vi "ReadBinaryCore.vi"(7 "UpperLevelControlRefs.":T1, 9 "metadata in":refnum<queue>, 10 "data out in":refnum<queue>, 11 "Control Queue in":refnum<queue>) -> ()   [LabVIEW 2013]
uses:
  _BinaryFileViewer/ReaderUpperLevelRefs.ctl
  _BinaryFileViewer/BinaryReader_Params.ctl
  ControlDef/ProcessingMode.ctl
  _BinaryFileViewer/BinaryRead_State.ctl
  Signal_Segment.ctl
  BinaryHeader.ctl
  Signal_Segment_v3.ctl
  Signal_Segment_v35.ctl
  Signal_Segment_v36.ctl
  _FileFormatConversion/UIC-DepthProfileFormat/DepthProfileFileHeader.ctl
  _FileFormatConversion/UIC-DepthProfileFormat/DepthProfileFormat_Spectrum.ctl
  <vilib>/Utility/error.llb/DialogType.ctl
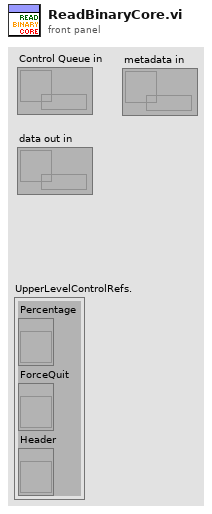
[diagram p1: front panel]
types:
  T1 = typedef "ReaderUpperLevelRefs.ctl" = cluster{"Percentage":refnum<vi>, "ForceQuit":refnum<vi>, "Header":refnum<vi>}
  T2 = typedef "BinaryReader_Params.ctl" = cluster{"FileVersion":string, "Start Position":dbl[], "StepWidth":dbl[], "Dimension":i32[], "TotalDepth":i32, "Spec#":u32, "FileSize":i64, "Calibr.":dbl[], "Position":dbl[], "Pressure":dbl, "Desp_LaserEnergy":dbl, "PI_LaserEnergy":dbl, "SpecLength":dbl, "Average#":i32, "SampleRate":dbl, "DAQ_Range":dbl, "Voltages Table":sgl[][], "ProcMode":T3, "Time Stamp":timestamp, "TrigDelay":dbl, "TickCount":dbl}
  T3 = typedef "ProcessingMode.ctl" = enum16{"None", "Drop by Threshold", "TDC Simulate", "SetFilter"}
  T4 = enum16{"open", "replace", "create", "open or create", "replace or create", "replace or create with confirmation"}
  T5 = typedef "Signal_Segment_v3.ctl" = cluster{"Signal":sgl[], "Calibr.":dbl[], "Position":dbl[], "Pressure":dbl, "Desp_LaserEnergy":dbl, "PI_LaserEnergy":dbl, "Depth":dbl, "Average":i32, "Acqu. Rate":dbl, "Voltages Table":sgl[][], "Acqu. Range":dbl, "Processing Mode":T3, "Threshold":dbl, "Comment":string, "Time Stamp":timestamp, "Operator":string}
  T6 = enum16{"big-endian, network order", "native, host order", "little-endian"}
  T7 = typedef "BinaryHeader.ctl" = cluster{"Start Position":dbl[], "StepWidth":dbl[], "Dimension":i32[], "SpecLength":i32}
  T8 = typedef "Signal_Segment_v35.ctl" = cluster{"SampleRate":dbl, "TrigDelay":dbl, "SpecLength":dbl, "DAQ_Range":dbl, "Average#":i32, "Position":dbl[], "Spectrum":sgl[], "Calibr.":dbl[], "Pressure":dbl, "Desp_LaserEnergy":dbl, "PI_LaserEnergy":dbl, "Voltages Table":sgl[][], "ProcMode":T3, "Threshold":dbl, "Comment":string, "Time Stamp":timestamp}
  T9 = typedef "Signal_Segment_v36.ctl" = cluster{"SampleRate":dbl, "TrigDelay":dbl, "SpecLength":dbl, "DAQ_Range":dbl, "Average#":i32, "Position":dbl[], "Spectrum":sgl[], "Calibr.":dbl[], "Pressure":dbl, "Desp_LaserEnergy":dbl, "PI_LaserEnergy":dbl, "Voltages Table":sgl[][], "ProcMode":T3, "Threshold":dbl, "Comment":string, "TickCount":dbl, "Time Stamp":timestamp}
  T10 = typedef "DepthProfileFormat_Spectrum.ctl" = cluster{"Average#":i16, "SpecLength":i32, "Spectrum":sgl[], "Cali.":dbl[], "Sample Rate":dbl}
  T11 = typedef "Signal_Segment.ctl" = cluster{"SampleRate":dbl, "TrigDelay":dbl, "SpecLength":dbl, "DAQ_Range":dbl, "Average#":i32, "Position":dbl[], "Spectrum":sgl[], "Calibr.":dbl[], "Pressure":dbl, "Desp_LaserEnergy":dbl, "PI_LaserEnergy":dbl, "Voltages Table":sgl[][], "ProcMode":T3, "Threshold":dbl, "Comment":string, "TickCount":dbl, "Time Stamp":timestamp}
  T12 = typedef "BinaryRead_State.ctl" = cluster{"State":enum16{"Open", "GetHeader", "Index", "Read_i", "Read_all", "Close", "Quit"}, "Params":variant}
  T13 = enum16{"Open", "GetHeader", "Index", "Read_i", "Read_all", "Close", "Quit"}
  T14 = typedef "DepthProfileFileHeader.ctl" = cluster{"SpecLength":i32, "Sample Rate":dbl, "Cali.":dbl[], "Total_Depth":i32}
  T15 = typedef "DialogType.ctl" = u16
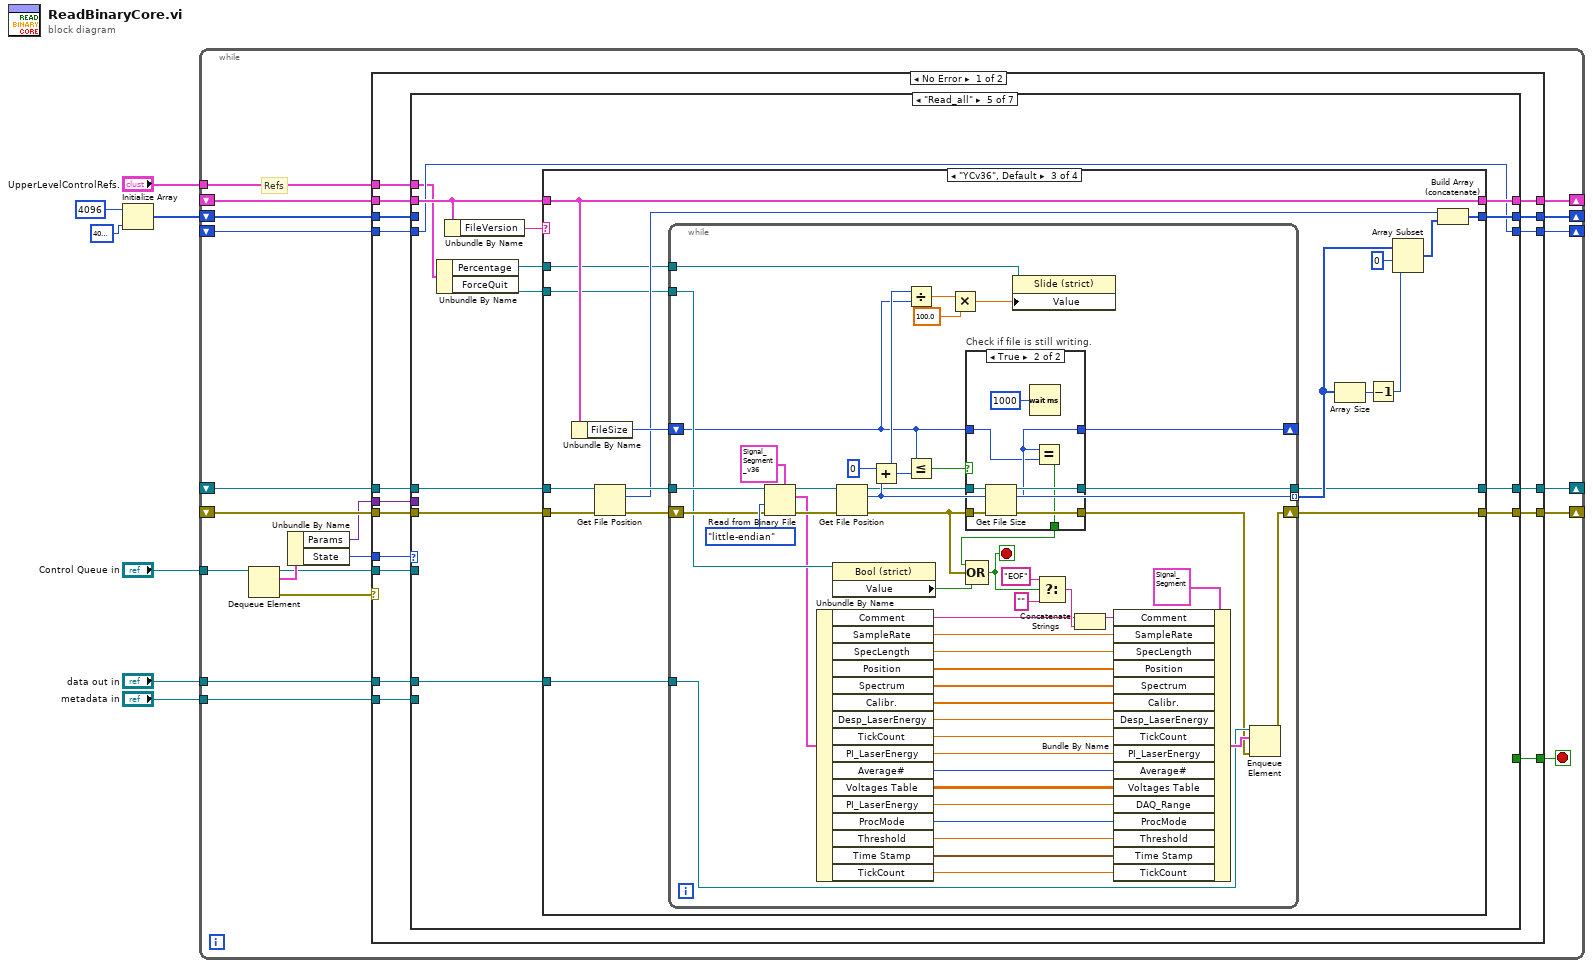
[diagram p0: block diagram]
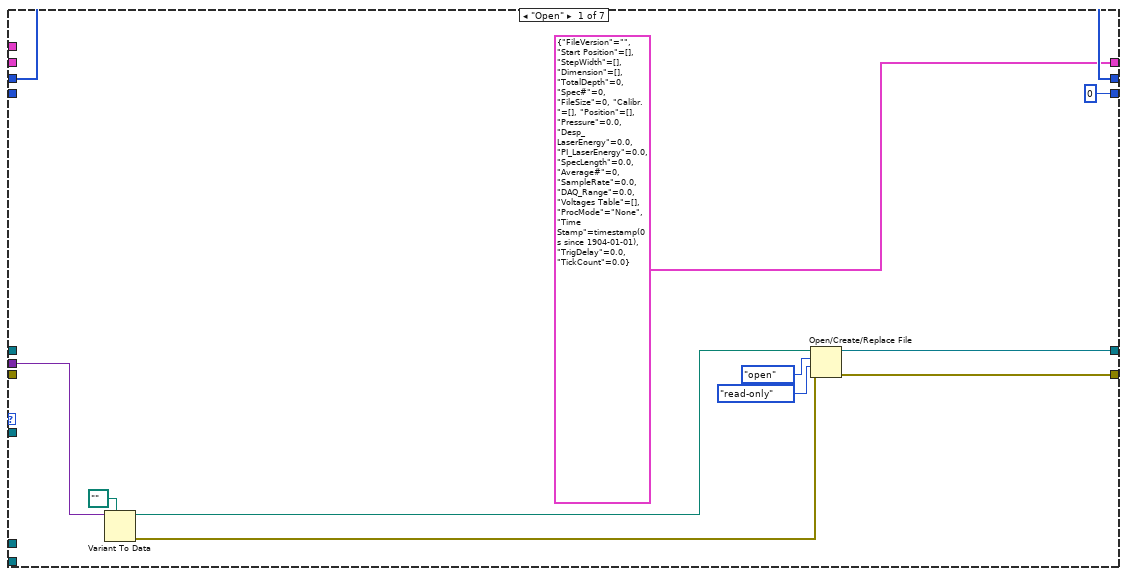
[diagram p2: hidden frame]
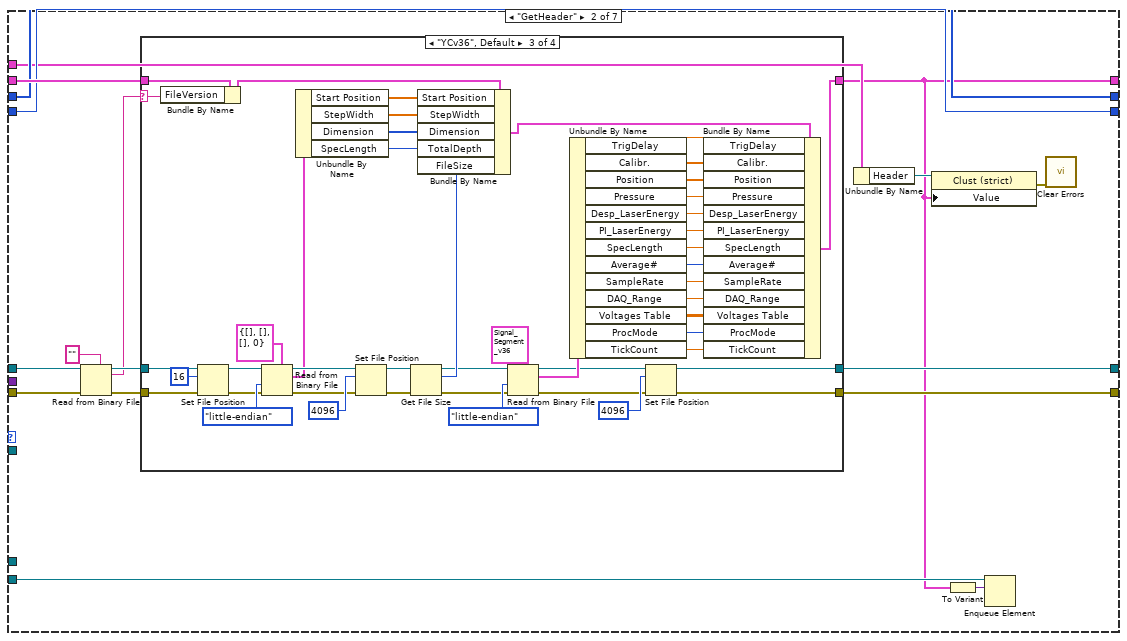
[diagram p3: hidden frame]
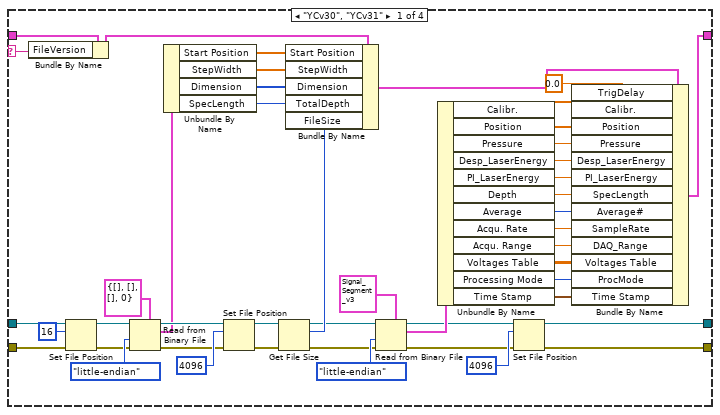
[diagram p4: hidden frame]
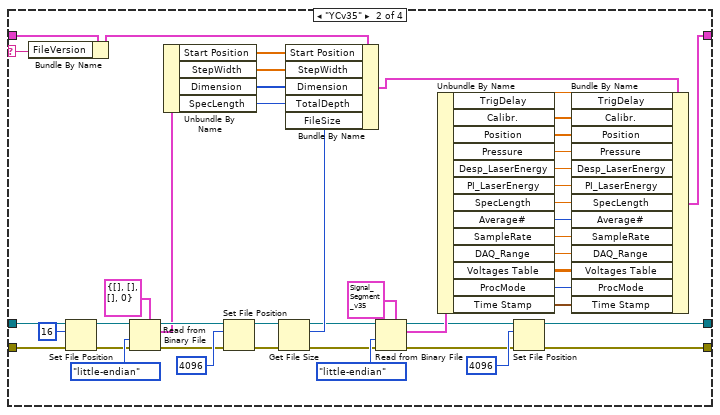
[diagram p5: hidden frame]
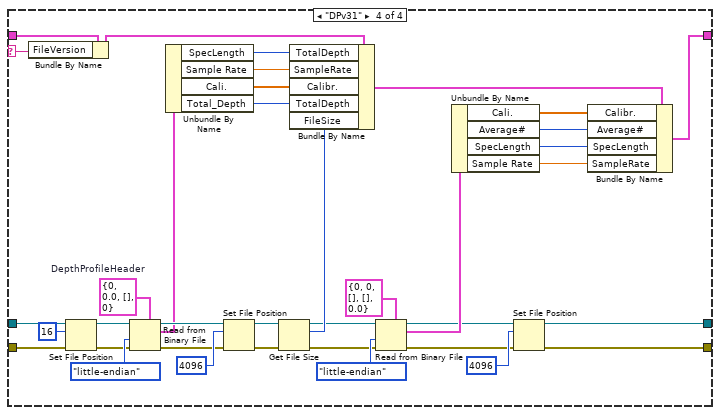
[diagram p6: hidden frame]
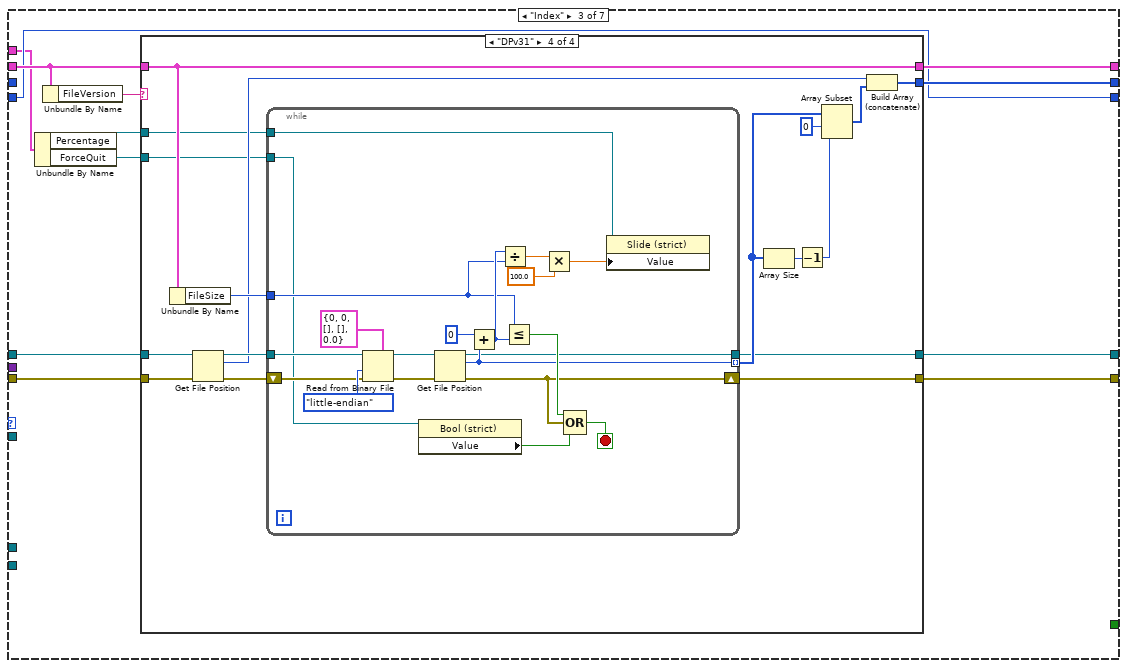
[diagram p7: hidden frame]
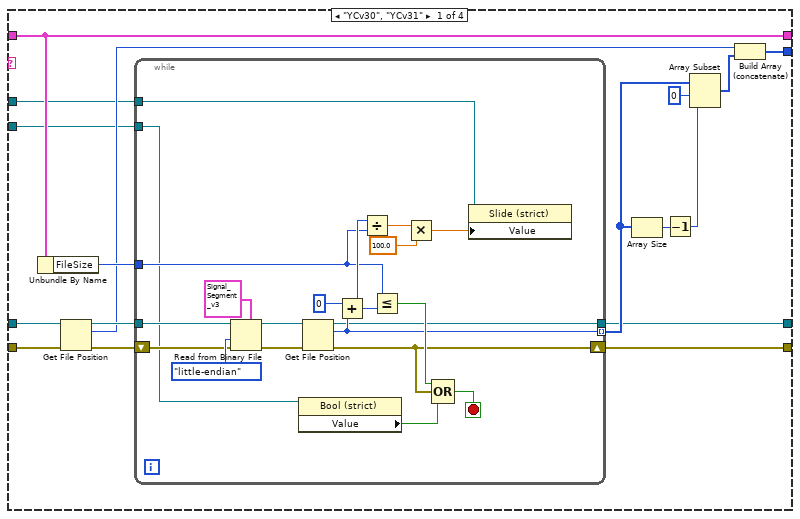
[diagram p8: hidden frame]
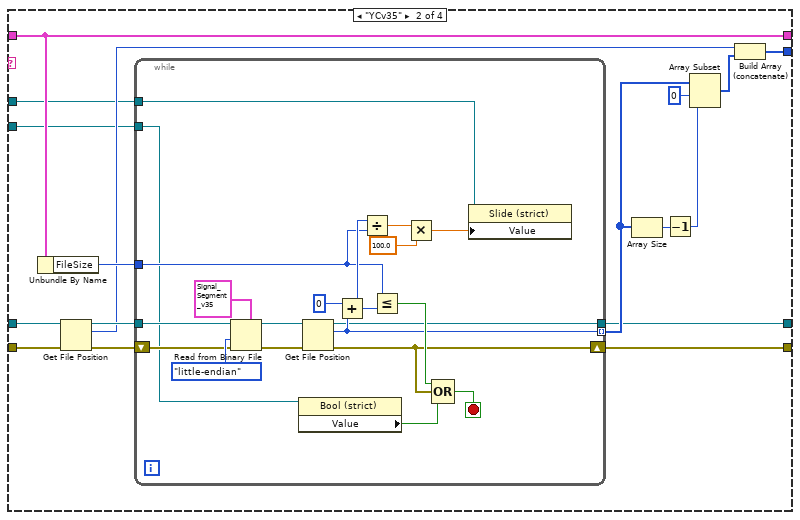
[diagram p9: hidden frame]
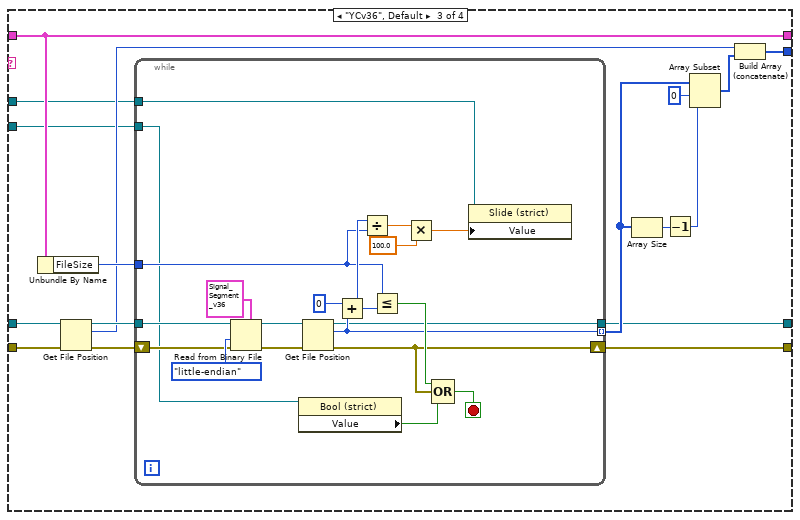
[diagram p10: hidden frame]
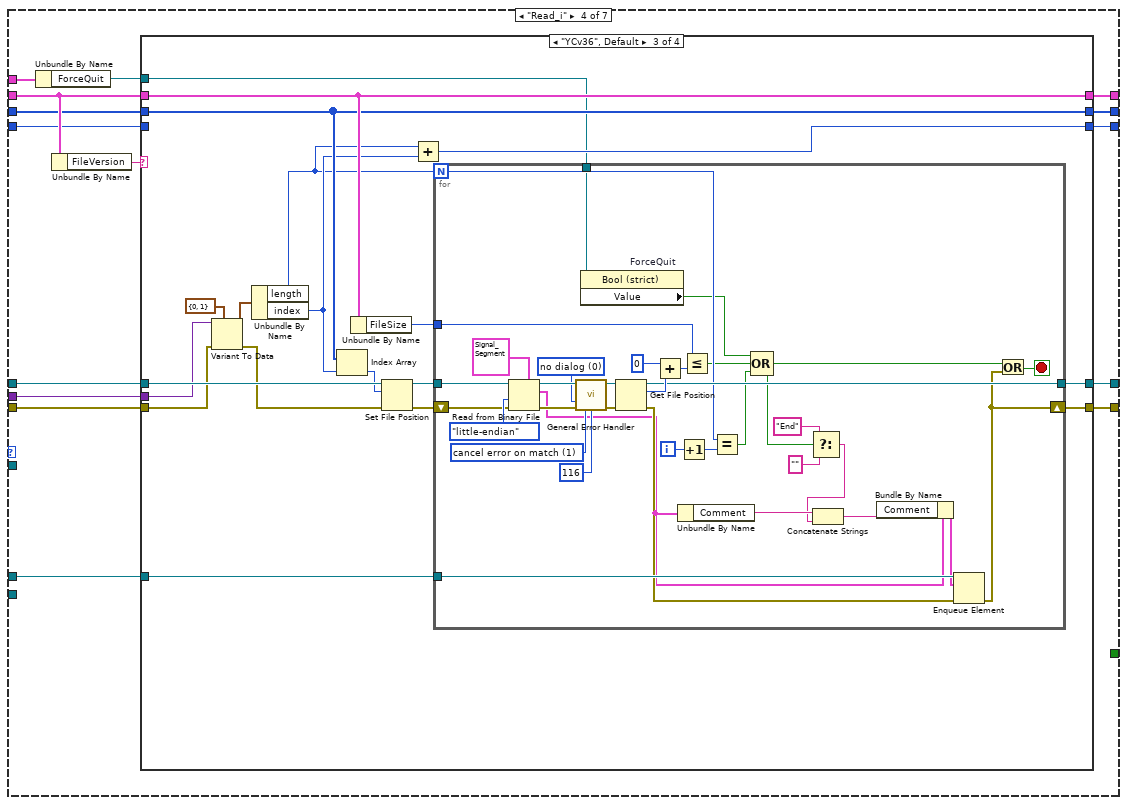
[diagram p11: hidden frame]
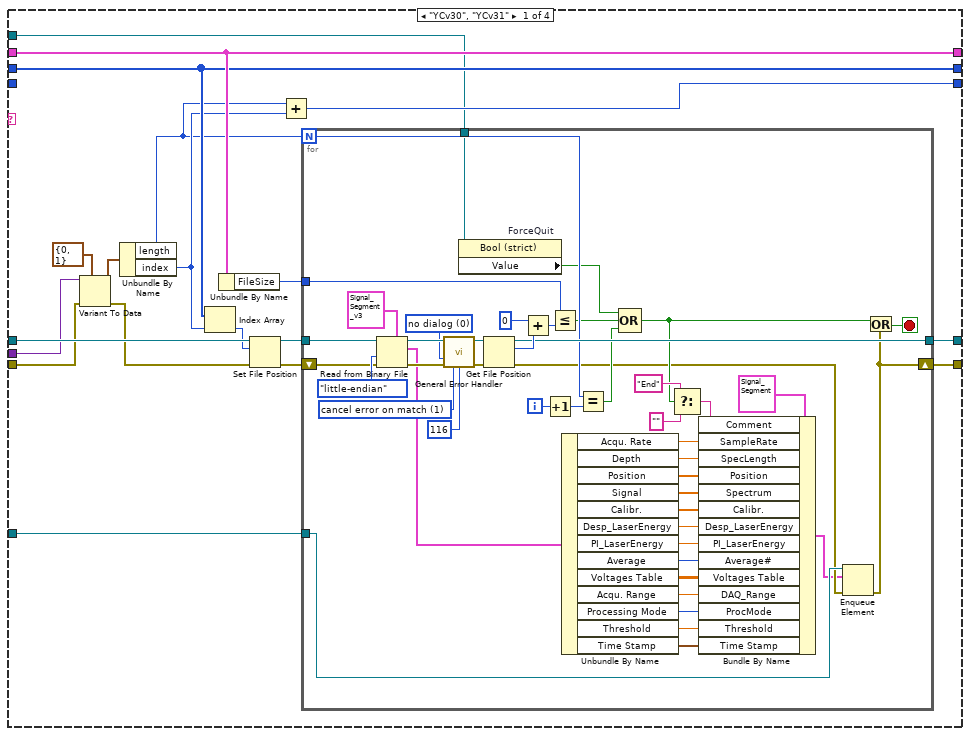
[diagram p12: hidden frame]
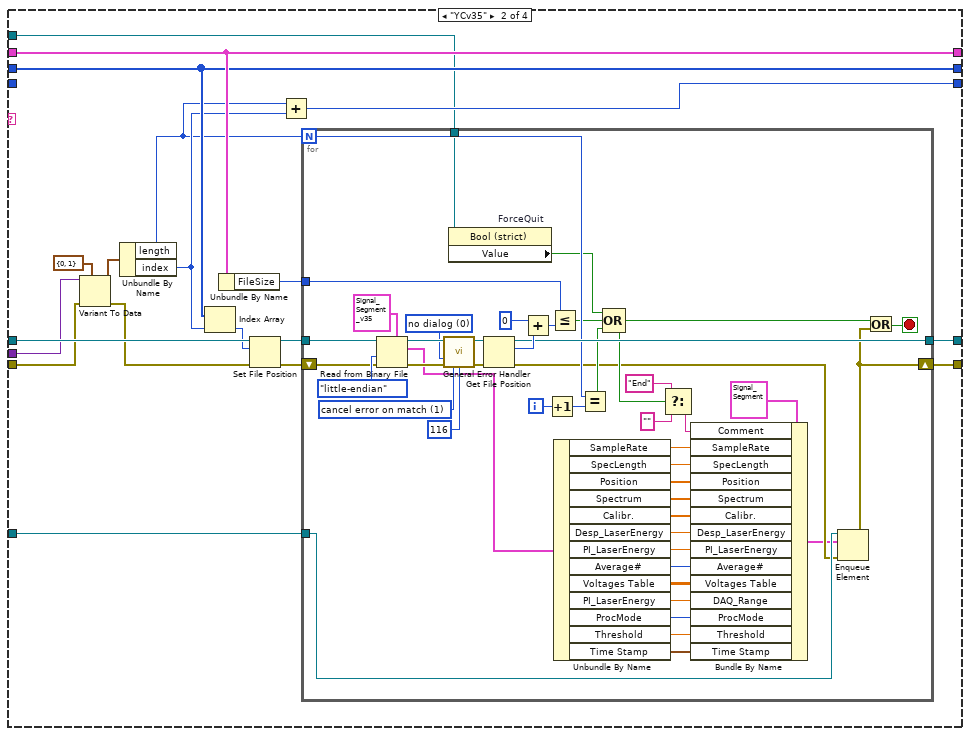
[diagram p13: hidden frame]
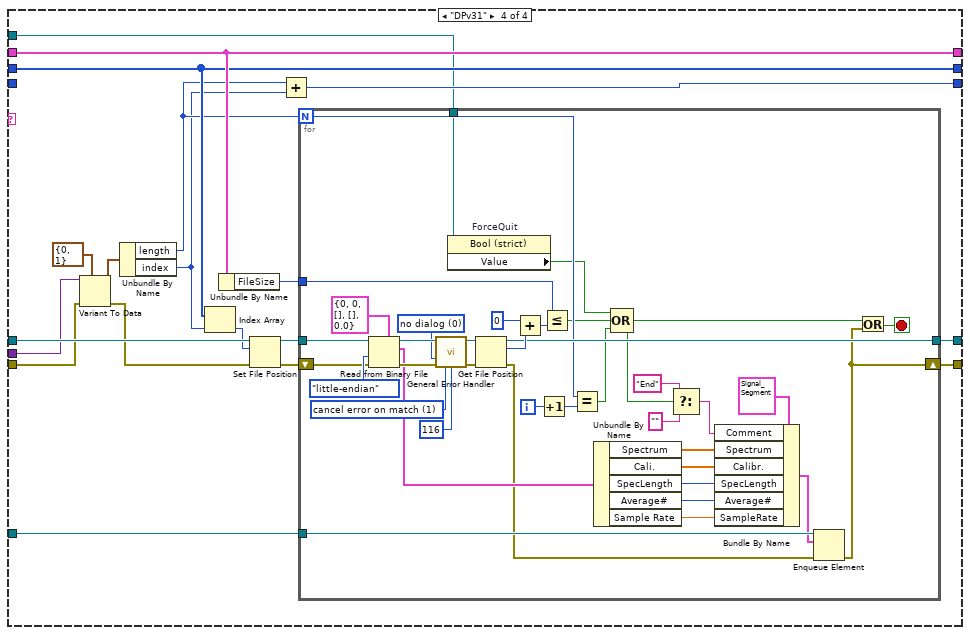
[diagram p14: hidden frame]
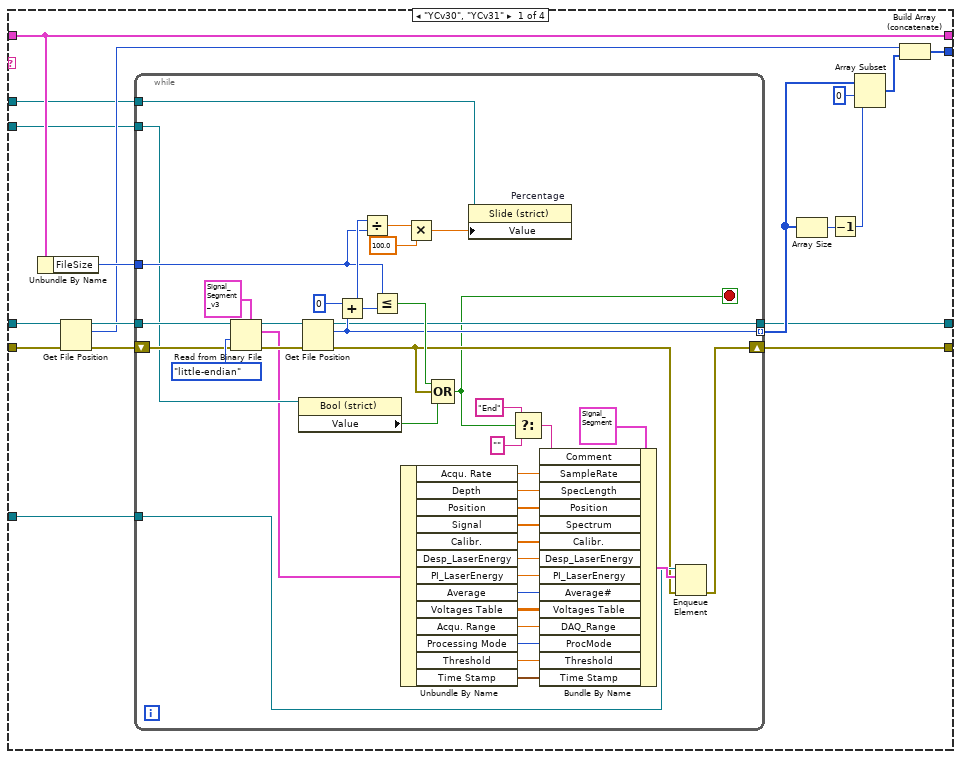
[diagram p15: hidden frame]
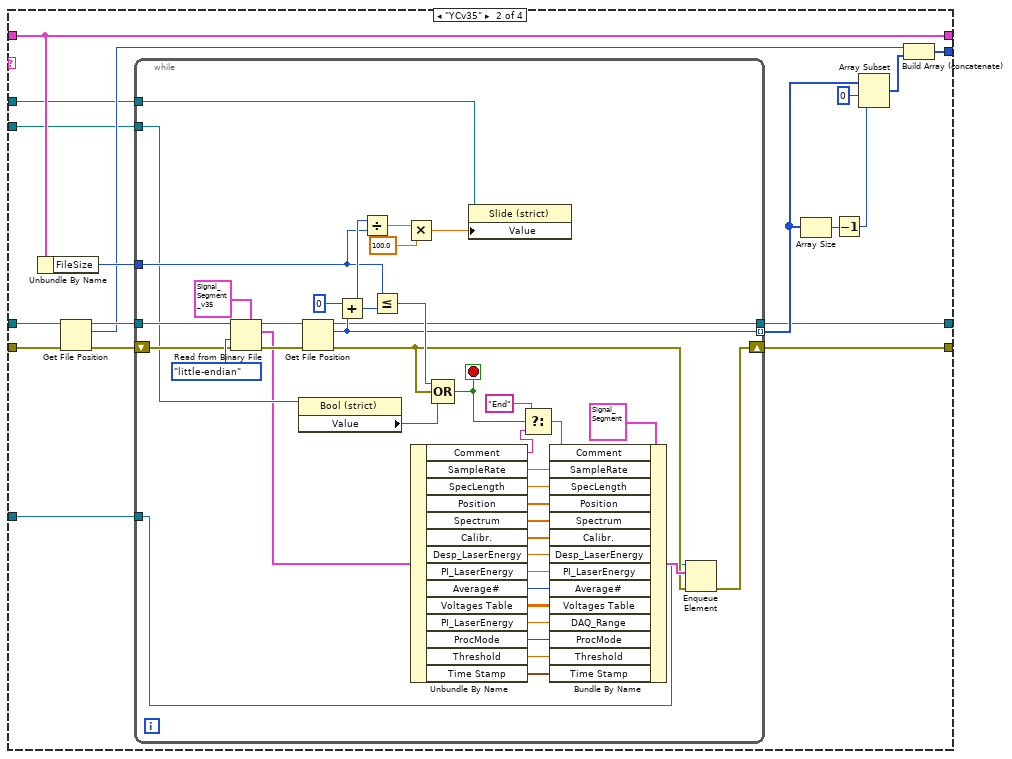
[diagram p16: hidden frame]
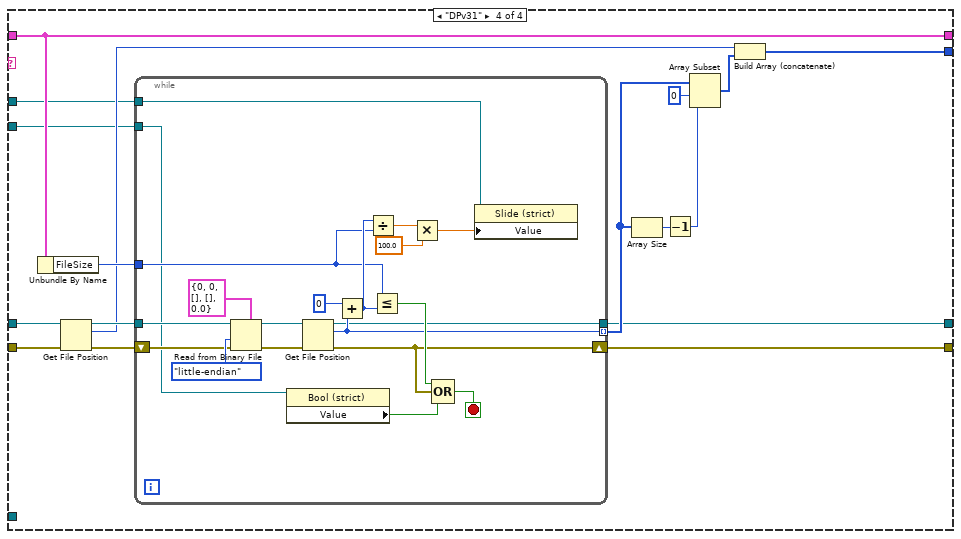
[diagram p18: hidden frame]
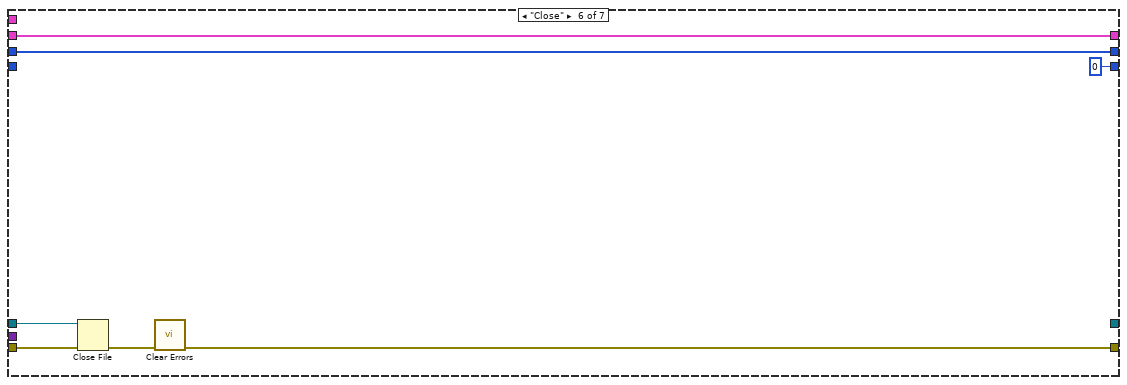
[diagram p19: hidden frame]
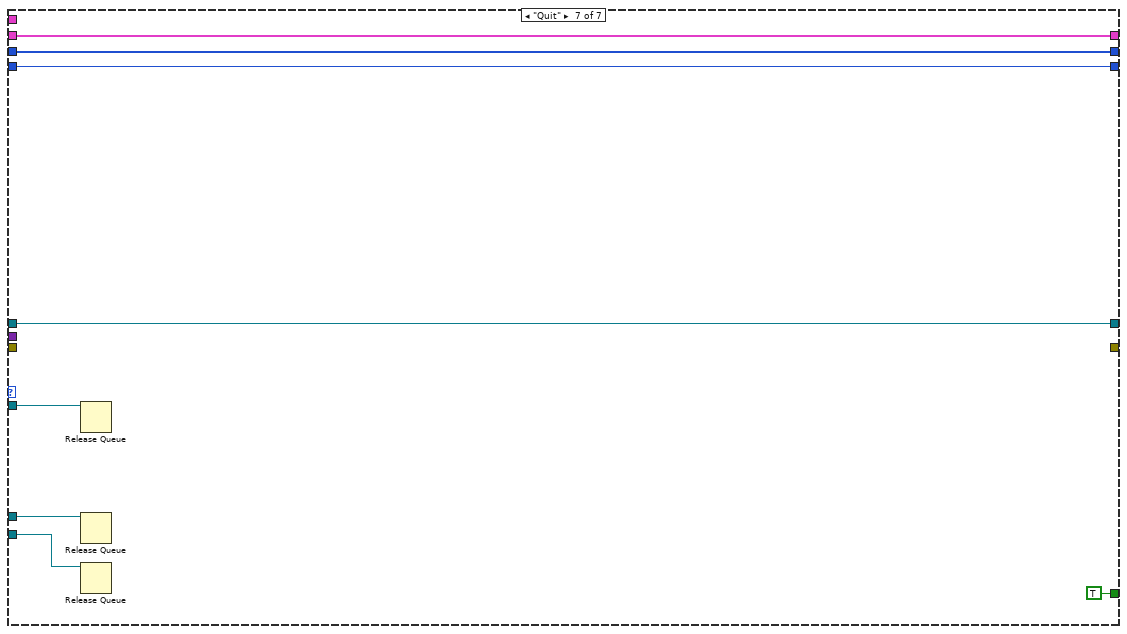
[diagram p20: hidden frame]
diagram:
  n1 = Initialize Array(i64 4096, 4000000 ("dimension size")) -> (w4:i64[])
  n2 = while {
    shift-right: [w26] -> _
    shift-left: _ -> [w27]
    shift-right: [w25] -> _
    shift-left: _ -> [w24]
    shift-right: [w23] -> _
    shift-left: _ -> [w22]
    shift-right: [w20] -> _
    shift-left: w4 -> [w21]
    tunnel: "data out in" -> [w19]
    shift-right: [w17] -> _
    shift-left: _ -> [w18]
    tunnel: "Control Queue in" -> [w16]
    tunnel: "UpperLevelControlRefs." -> [w10]
    tunnel: "metadata in" -> [w9]
    stop <- w11 stop-if-true
    # "Refs"
    n3 = Dequeue Element(queue=w16) -> (queue out=w8:refnum<queue>, element=w15:T12, error out=w12:errorcluster)  [unwired: 2 in, 1 out]
    n4 = Unbundle By Name(w15) -> ("Params"=w13:variant, "State"=w14:T13)
    n5 = case shown="No Error" w12 {
      tunnel: w27 -> [w44 w925]
      tunnel: [w43 w925] -> w26
      tunnel: [w42 w926] -> w25
      tunnel: w24 -> [w41 w926]
      tunnel: [w40 w929] -> w23
      tunnel: w22 -> [w39 w929]
      tunnel: w21 -> [w38 w928]
      tunnel: [w37 w928] -> w20
      tunnel: w19 -> [w36 _]
      tunnel: w18 -> [w35 w927]
      tunnel: [w34 w927] -> w17
      tunnel: w14 -> [w33 _]
      tunnel: w13 -> [w32 _]
      tunnel: [w31 TRUE] -> w11
      tunnel: w10 -> [w30 _]
      tunnel: w9 -> [w29 _]
      tunnel: w8 -> [w28 _]
      frame No Error {
        n6 = case shown="\"Read_all\"" w33 {
          tunnel: w44 -> [_ w72 w255 w419 w671 w911 _]
          tunnel: [w46 w66 w259 w410 w675 w910 _] -> w43
          tunnel: [w47 w65 w258 w422 w674 _ w923] -> w42
          tunnel: w41 -> [_ w69 w256 w420 w672 w915 w923]
          tunnel: [T2 {"FileVersion"="", "Start Position"=[], "StepWidth"=[], "Dimension"=[], "TotalDepth"=0, "Spec#"=0, "FileSize"=0, "Calibr."=[], "Position"=[], "Pressure"=0.0, "Desp_LaserEnergy"=0.0, "PI_LaserEnergy"=0.0, "SpecLength"=0.0, "Average#"=0, "SampleRate"=0.0, "DAQ_Range"=0.0, "Voltages Table"=[], "ProcMode"=enum."None", "Time Stamp"=timestamp(0 s since 1904-01-01), "TrigDelay"=0.0, "TickCount"=0.0} ("Header") w56 w257 w421 w673 w914 w922] -> w40
          tunnel: w39 -> [_ w64 w254 w418 w670 w914 w922]
          tunnel: w38 -> [w48 w63 _ w415 _ w913 w921]
          tunnel: [w48 w63 w252 w416 w668 w913 w921] -> w37
          tunnel: w32 -> [w52 _ _ w414 _ _ _]
          tunnel: w36 -> [_ _ _ w413 w663 _ w919]
          tunnel: w35 -> [_ w62 w251 w412 w667 _ w920]
          tunnel: [0 ("index") w62 w251 w411 w667 0 ("index") w920] -> w34
          tunnel: [_ _ _ _ _ _ TRUE] -> w31
          tunnel: w30 -> [_ w61 w250 w409 w666 _ _]
          tunnel: w29 -> [_ w59 _ _ _ _ w917]
          tunnel: w28 -> [_ _ _ _ _ _ w916]
          frame "Open" {
            n7 = Variant To Data(type=path "" ("file path (use dialog)"), Variant=w52) -> (data=w51:path, error out=w50:errorcluster)  [unwired: 1 in]
            n8 = Open/Create/Replace File(file path (use dialog)=w51, error in=w50, operation (0:open)=T4."open", access (0:read/write)=enum16{"read/write", "read-only", "write-only"}."read-only") -> (refnum out=w47:refnum<file>, error out=w46:errorcluster)  [unwired: 2 in, 1 out]
          }
          frame "GetHeader" {
            n9 = Read from Binary File(5:"" ("data type"), 8:w72, 11:w69) -> (0:w71:errorcluster, 2:w68:string, 3:w70:refnum<file>)  [unwired: 3 in, 1 out]
            n10 = case shown="\"YCv36\", Default" w68 {
              selector: w68 -> [w100 w146 w192 w230]
              tunnel: w71 -> [w113 w159 w205 w243]
              tunnel: w70 -> [w112 w158 w204 w242]
              tunnel: [w75 w122 w168 w215] -> w66
              tunnel: [w76 w123 w169 w216] -> w65
              tunnel: [w91 w137 w183 w222] -> w56
              tunnel: w64 -> [w108 w154 w200 w238]
              frame "YCv30", "YCv31" {
                n11 = Bundle By Name(cluster=w108, "FileVersion"=w100) -> (w101:T2)
                n12 = Set File Position(offset (in bytes) (0)=i64 16, refnum=w112, error in=w113) -> (refnum out=w116:refnum<file>, error out=w114:errorcluster)  [unwired: 1 in]
                n13 = Read from Binary File(5:T7 {"Start Position"=[], "StepWidth"=[], "Dimension"=[], "SpecLength"=0} ("File Header"), 8:w114, 9:T6."little-endian" ("byte order (0:big-endian, network order)"), 11:w116) -> (0:w96:errorcluster, 2:w106:T7, 3:w110:refnum<file>)  [unwired: 2 in, 1 out]
                n14 = Unbundle By Name(w106) -> ("Start Position"=w105:dbl[], "StepWidth"=w104:dbl[], "Dimension"=w103:i32[], "SpecLength"=w102:i32)
                n15 = Set File Position(offset (in bytes) (0)=i64 4096, refnum=w110, error in=w96) -> (refnum out=w111:refnum<file>, error out=w95:errorcluster)  [unwired: 1 in]
                n16 = Get File Size(file=w111, error in=w95) -> (refnum out=w93:refnum<file>, size (in bytes)=w99:i64, 0:w94:errorcluster)
                n17 = Bundle By Name(cluster=w101, "Start Position"=w105, "StepWidth"=w104, "Dimension"=w103, "TotalDepth"=w102, "FileSize"=w99) -> (w107:T2)
                n18 = Read from Binary File(5:T5 {"Signal"=[], "Calibr."=[], "Position"=[], "Pressure"=0.0, "Desp_LaserEnergy"=0.05, "PI_LaserEnergy"=0.05, "Depth"=0.0, "Average"=0, "Acqu. Rate"=0.0, "Voltages Table"=[], "Acqu. Range"=0.0, "Processing Mode"=enum."None", "Threshold"=0.05, "Comment"="", "Time Stamp"=timestamp(0 s since 1904-01-01), "Operator"=""} ("Signal Segment"), 8:w94, 9:T6."little-endian" ("byte order (0:big-endian, network order)"), 11:w93) -> (0:w74:errorcluster, 2:w92:T5, 3:w77:refnum<file>)  [unwired: 2 in, 1 out]
                n19 = Unbundle By Name(w92) -> ("Calibr."=w90:dbl[], "Position"=w89:dbl[], "Pressure"=w88:dbl, "Desp_LaserEnergy"=w87:dbl, "PI_LaserEnergy"=w86:dbl, "Depth"=w85:dbl, "Average"=w84:i32, "Acqu. Rate"=w83:dbl, "Acqu. Range"=w82:dbl, "Voltages Table"=w81:sgl[][], "Processing Mode"=w80:T3, "Time Stamp"=w79:timestamp)
                n20 = Set File Position(offset (in bytes) (0)=i64 4096, refnum=w77, error in=w74) -> (refnum out=w76:refnum<file>, error out=w75:errorcluster)  [unwired: 1 in]
                n21 = Bundle By Name(cluster=w107, "TrigDelay"=0.0, "Calibr."=w90, "Position"=w89, "Pressure"=w88, "Desp_LaserEnergy"=w87, "PI_LaserEnergy"=w86, "SpecLength"=w85, "Average#"=w84, "SampleRate"=w83, "DAQ_Range"=w82, "Voltages Table"=w81, "ProcMode"=w80, "Time Stamp"=w79) -> (w91:T2)
              }
              frame "YCv35" {
                n22 = Bundle By Name(cluster=w154, "FileVersion"=w146) -> (w147:T2)
                n23 = Set File Position(offset (in bytes) (0)=i64 16, refnum=w158, error in=w159) -> (refnum out=w162:refnum<file>, error out=w160:errorcluster)  [unwired: 1 in]
                n24 = Read from Binary File(5:T7 {"Start Position"=[], "StepWidth"=[], "Dimension"=[], "SpecLength"=0} ("File Header"), 8:w160, 9:T6."little-endian" ("byte order (0:big-endian, network order)"), 11:w162) -> (0:w142:errorcluster, 2:w152:T7, 3:w156:refnum<file>)  [unwired: 2 in, 1 out]
                n25 = Unbundle By Name(w152) -> ("Start Position"=w151:dbl[], "StepWidth"=w150:dbl[], "Dimension"=w149:i32[], "SpecLength"=w148:i32)
                n26 = Set File Position(offset (in bytes) (0)=i64 4096, refnum=w156, error in=w142) -> (refnum out=w157:refnum<file>, error out=w141:errorcluster)  [unwired: 1 in]
                n27 = Get File Size(file=w157, error in=w141) -> (refnum out=w139:refnum<file>, size (in bytes)=w145:i64, 0:w140:errorcluster)
                n28 = Bundle By Name(cluster=w147, "Start Position"=w151, "StepWidth"=w150, "Dimension"=w149, "TotalDepth"=w148, "FileSize"=w145) -> (w153:T2)
                n29 = Read from Binary File(5:T8 {"SampleRate"=0.0, "TrigDelay"=0.0, "SpecLength"=0.0, "DAQ_Range"=0.0, "Average#"=0, "Position"=[], "Spectrum"=[], "Calibr."=[], "Pressure"=0.0, "Desp_LaserEnergy"=0.0, "PI_LaserEnergy"=0.0, "Voltages Table"=[], "ProcMode"=enum."None", "Threshold"=0.0, "Comment"="", "Time Stamp"=timestamp(0 s since 1904-01-01)} ("Signal Segment"), 8:w140, 9:T6."little-endian" ("byte order (0:big-endian, network order)"), 11:w139) -> (0:w121:errorcluster, 2:w138:T8, 3:w124:refnum<file>)  [unwired: 2 in, 1 out]
                n30 = Unbundle By Name(w138) -> ("TrigDelay"=w120:dbl, "Calibr."=w136:dbl[], "Position"=w135:dbl[], "Pressure"=w134:dbl, "Desp_LaserEnergy"=w133:dbl, "PI_LaserEnergy"=w132:dbl, "SpecLength"=w131:dbl, "Average#"=w130:i32, "SampleRate"=w129:dbl, "DAQ_Range"=w128:dbl, "Voltages Table"=w127:sgl[][], "ProcMode"=w126:T3, "Time Stamp"=w119:timestamp)
                n31 = Set File Position(offset (in bytes) (0)=i64 4096, refnum=w124, error in=w121) -> (refnum out=w123:refnum<file>, error out=w122:errorcluster)  [unwired: 1 in]
                n32 = Bundle By Name(cluster=w153, "TrigDelay"=w120, "Calibr."=w136, "Position"=w135, "Pressure"=w134, "Desp_LaserEnergy"=w133, "PI_LaserEnergy"=w132, "SpecLength"=w131, "Average#"=w130, "SampleRate"=w129, "DAQ_Range"=w128, "Voltages Table"=w127, "ProcMode"=w126, "Time Stamp"=w119) -> (w137:T2)
              }
              frame "YCv36", Default {
                n33 = Bundle By Name(cluster=w200, "FileVersion"=w192) -> (w193:T2)
                n34 = Set File Position(offset (in bytes) (0)=i64 16, refnum=w204, error in=w205) -> (refnum out=w208:refnum<file>, error out=w206:errorcluster)  [unwired: 1 in]
                n35 = Read from Binary File(5:T7 {"Start Position"=[], "StepWidth"=[], "Dimension"=[], "SpecLength"=0} ("File Header"), 8:w206, 9:T6."little-endian" ("byte order (0:big-endian, network order)"), 11:w208) -> (0:w188:errorcluster, 2:w198:T7, 3:w202:refnum<file>)  [unwired: 2 in, 1 out]
                n36 = Unbundle By Name(w198) -> ("Start Position"=w197:dbl[], "StepWidth"=w196:dbl[], "Dimension"=w195:i32[], "SpecLength"=w194:i32)
                n37 = Set File Position(offset (in bytes) (0)=i64 4096, refnum=w202, error in=w188) -> (refnum out=w203:refnum<file>, error out=w187:errorcluster)  [unwired: 1 in]
                n38 = Get File Size(file=w203, error in=w187) -> (refnum out=w185:refnum<file>, size (in bytes)=w191:i64, 0:w186:errorcluster)
                n39 = Bundle By Name(cluster=w193, "Start Position"=w197, "StepWidth"=w196, "Dimension"=w195, "TotalDepth"=w194, "FileSize"=w191) -> (w199:T2)
                n40 = Read from Binary File(5:T9 {"SampleRate"=-1.0, "TrigDelay"=0.0, "SpecLength"=0.0, "DAQ_Range"=0.0, "Average#"=0, "Position"=[], "Spectrum"=[], "Calibr."=[], "Pressure"=-1.0, "Desp_LaserEnergy"=-1.0, "PI_LaserEnergy"=-1.0, "Voltages Table"=[], "ProcMode"=enum."None", "Threshold"=-1.0, "Comment"="", "TickCount"=0.0, "Time Stamp"=timestamp(0 s since 1904-01-01)} ("Signal Segment"), 8:w186, 9:T6."little-endian" ("byte order (0:big-endian, network order)"), 11:w185) -> (0:w167:errorcluster, 2:w184:T9, 3:w170:refnum<file>)  [unwired: 2 in, 1 out]
                n41 = Unbundle By Name(w184) -> ("TrigDelay"=w166:dbl, "Calibr."=w182:dbl[], "Position"=w181:dbl[], "Pressure"=w180:dbl, "Desp_LaserEnergy"=w179:dbl, "PI_LaserEnergy"=w178:dbl, "SpecLength"=w177:dbl, "Average#"=w176:i32, "SampleRate"=w175:dbl, "DAQ_Range"=w174:dbl, "Voltages Table"=w173:sgl[][], "ProcMode"=w172:T3, "TickCount"=w165:dbl)
                n42 = Set File Position(offset (in bytes) (0)=i64 4096, refnum=w170, error in=w167) -> (refnum out=w169:refnum<file>, error out=w168:errorcluster)  [unwired: 1 in]
                n43 = Bundle By Name(cluster=w199, "TrigDelay"=w166, "Calibr."=w182, "Position"=w181, "Pressure"=w180, "Desp_LaserEnergy"=w179, "PI_LaserEnergy"=w178, "SpecLength"=w177, "Average#"=w176, "SampleRate"=w175, "DAQ_Range"=w174, "Voltages Table"=w173, "ProcMode"=w172, "TickCount"=w165) -> (w183:T2)
              }
              frame "DPv31" {
                w213 = T14 {"SpecLength"=0, "Sample Rate"=0.0, "Cali."=[], "Total_Depth"=0}  # DepthProfileHeader
                n44 = Bundle By Name(cluster=w238, "FileVersion"=w230) -> (w231:T2)
                n45 = Set File Position(offset (in bytes) (0)=i64 16, refnum=w242, error in=w243) -> (refnum out=w246:refnum<file>, error out=w244:errorcluster)  [unwired: 1 in]
                n46 = Read from Binary File(5:w213, 8:w244, 9:T6."little-endian" ("byte order (0:big-endian, network order)"), 11:w246) -> (0:w227:errorcluster, 2:w236:T14, 3:w240:refnum<file>)  [unwired: 2 in, 1 out]
                n47 = Unbundle By Name(w236) -> ("SpecLength"=w235:i32, "Sample Rate"=w234:dbl, "Cali."=w233:dbl[], "Total_Depth"=w232:i32)
                n48 = Set File Position(offset (in bytes) (0)=i64 4096, refnum=w240, error in=w227) -> (refnum out=w241:refnum<file>, error out=w226:errorcluster)  [unwired: 1 in]
                n49 = Get File Size(file=w241, error in=w226) -> (refnum out=w224:refnum<file>, size (in bytes)=w229:i64, 0:w225:errorcluster)
                n50 = Bundle By Name(cluster=w231, "TotalDepth"=w235, "SampleRate"=w234, "Calibr."=w233, "TotalDepth"=w232, "FileSize"=w229) -> (w237:T2)
                n51 = Read from Binary File(5:T10 {"Average#"=0, "SpecLength"=0, "Spectrum"=[], "Cali."=[], "Sample Rate"=0.0} ("cluster"), 8:w225, 9:T6."little-endian" ("byte order (0:big-endian, network order)"), 11:w224) -> (0:w214:errorcluster, 2:w223:T10, 3:w217:refnum<file>)  [unwired: 2 in, 1 out]
                n52 = Unbundle By Name(w223) -> ("Cali."=w221:dbl[], "Average#"=w220:i16, "SpecLength"=w219:i32, "Sample Rate"=w211:dbl)
                n53 = Set File Position(offset (in bytes) (0)=i64 4096, refnum=w217, error in=w214) -> (refnum out=w216:refnum<file>, error out=w215:errorcluster)  [unwired: 1 in]
                n54 = Bundle By Name(cluster=w237, "Calibr."=w221, "Average#"=w220, "SpecLength"=w219, "SampleRate"=w211) -> (w222:T2)
              }
            }
            n55 = Unbundle By Name(w61) -> ("Header"=w60:refnum<vi>)
            n56 = property class="Clust (strict)"(reference=w60, "Value"=w56) -> (error out=w58:errorcluster)  [unwired: 1 in, 1 out]
            n57 = To Variant(anything=w56) -> (Variant=w57:variant)
            n58 = Enqueue Element(queue=w59, element=w57) -> ()  [unwired: 2 in, 3 out]
            n59 = call <vilib>:"Clear Errors.vi"("error in (no error)"=w58) -> ()  [unwired: 6 in, 1 out]
          }
          frame "Index" {
            n60 = Unbundle By Name(w250) -> ("Percentage"=w249:refnum<vi>, "ForceQuit"=w248:refnum<vi>)
            n61 = Unbundle By Name(w254) -> ("FileVersion"=w253:string)
            n62 = case shown="\"DPv31\"" w253 {
              tunnel: w255 -> [w275 w312 w349 w386]
              tunnel: w256 -> [w276 w313 w350 w387]
              tunnel: [w274 w311 w348 w385] -> w259
              tunnel: [w262 w299 w336 w373] -> w258
              tunnel: [w272 w309 w346 w383] -> w257
              tunnel: w254 -> [w272 w309 w346 w383]
              tunnel: [w269 w306 w343 w380] -> w252
              tunnel: w249 -> [w261 w298 w335 w372]
              tunnel: w248 -> [w260 w297 w334 w371]
              frame "YCv30", "YCv31" {
                n63 = Unbundle By Name(w272) -> ("FileSize"=w270:i64)
                n64 = Get File Position(4:w275, 7:w276) -> (0:w273:errorcluster, 2:w268:i64, 3:w271:refnum<file>)
                n65 = while {
                  tunnel: w271 -> [w290]
                  shift-right: [w287] -> w274
                  shift-left: w273 -> [w293]
                  tunnel: w270 -> [w279]
                  tunnel: [w286] -> w266 mode=indexing
                  tunnel: [w285] -> w262
                  tunnel: w261 -> [w281]
                  tunnel: w260 -> [w277]
                  stop <- w289 stop-if-true
                  n66 = Read from Binary File(5:T5 {"Signal"=[], "Calibr."=[], "Position"=[], "Pressure"=0.0, "Desp_LaserEnergy"=0.05, "PI_LaserEnergy"=0.05, "Depth"=0.0, "Average"=0, "Acqu. Rate"=0.0, "Voltages Table"=[], "Acqu. Range"=0.0, "Processing Mode"=enum."None", "Threshold"=0.05, "Comment"="", "Time Stamp"=timestamp(0 s since 1904-01-01), "Operator"=""} ("Signal Segment"), 8:w293, 9:T6."little-endian" ("byte order (0:big-endian, network order)"), 11:w290) -> (0:w294:errorcluster, 3:w291:refnum<file>)  [unwired: 2 in, 2 out]
                  n67 = property class="Bool (strict)"(reference=w277) -> ("Value"=w278:bool)  [unwired: 1 in, 2 out]
                  n68 = Get File Position(4:w294, 7:w291) -> (0:w287:errorcluster, 2:w286:i64, 3:w285:refnum<file>)
                  n69 = Add(x=i64 0, y=w286) -> (x+y=w280:i64)
                  n70 = Divide(x=w280, y=w279) -> (x/y=w283:dbl)
                  n71 = Less Or Equal?(x=w279, y=w280) -> (x <= y?=w288:bool)
                  n72 = Multiply(x=w283, y=100.0 ("x")) -> (x*y=w282:dbl)
                  n73 = Compound Arithmetic op=OR(w288, w287, w278) -> (w289:bool)
                  n74 = property class="Slide (strict)"(reference=w281, "Value"=w282) -> ()  [unwired: 1 in, 2 out]
                }
                n75 = Array Size(array=w266) -> (size(s)=w265:i32)
                n76 = Decrement(x=w265) -> (x-1=w264:i32)
                n77 = Array Subset(array=w266, index=0, length=w264) -> (w267:i64[])
                n78 = Build Array (concatenate)(w268, w267) -> (w269:i64[])
              }
              frame "YCv35" {
                n79 = Unbundle By Name(w309) -> ("FileSize"=w307:i64)
                n80 = Get File Position(4:w312, 7:w313) -> (0:w310:errorcluster, 2:w305:i64, 3:w308:refnum<file>)
                n81 = while {
                  tunnel: w308 -> [w327]
                  shift-right: [w324] -> w311
                  shift-left: w310 -> [w330]
                  tunnel: w307 -> [w316]
                  tunnel: [w323] -> w303 mode=indexing
                  tunnel: [w322] -> w299
                  tunnel: w298 -> [w318]
                  tunnel: w297 -> [w314]
                  stop <- w326 stop-if-true
                  n82 = Read from Binary File(5:T8 {"SampleRate"=-1.0, "TrigDelay"=0.0, "SpecLength"=0.0, "DAQ_Range"=0.0, "Average#"=0, "Position"=[], "Spectrum"=[], "Calibr."=[], "Pressure"=-1.0, "Desp_LaserEnergy"=-1.0, "PI_LaserEnergy"=-1.0, "Voltages Table"=[], "ProcMode"=enum."None", "Threshold"=-1.0, "Comment"="", "Time Stamp"=timestamp(0 s since 1904-01-01)} ("Signal Segment"), 8:w330, 9:T6."little-endian" ("byte order (0:big-endian, network order)"), 11:w327) -> (0:w331:errorcluster, 3:w328:refnum<file>)  [unwired: 2 in, 2 out]
                  n83 = property class="Bool (strict)"(reference=w314) -> ("Value"=w315:bool)  [unwired: 1 in, 2 out]
                  n84 = Get File Position(4:w331, 7:w328) -> (0:w324:errorcluster, 2:w323:i64, 3:w322:refnum<file>)
                  n85 = Add(x=i64 0, y=w323) -> (x+y=w317:i64)
                  n86 = Divide(x=w317, y=w316) -> (x/y=w320:dbl)
                  n87 = Less Or Equal?(x=w316, y=w317) -> (x <= y?=w325:bool)
                  n88 = Multiply(x=w320, y=100.0 ("x")) -> (x*y=w319:dbl)
                  n89 = Compound Arithmetic op=OR(w325, w324, w315) -> (w326:bool)
                  n90 = property class="Slide (strict)"(reference=w318, "Value"=w319) -> ()  [unwired: 1 in, 2 out]
                }
                n91 = Array Size(array=w303) -> (size(s)=w302:i32)
                n92 = Decrement(x=w302) -> (x-1=w301:i32)
                n93 = Array Subset(array=w303, index=0, length=w301) -> (w304:i64[])
                n94 = Build Array (concatenate)(w305, w304) -> (w306:i64[])
              }
              frame "YCv36", Default {
                n95 = Unbundle By Name(w346) -> ("FileSize"=w344:i64)
                n96 = Get File Position(4:w349, 7:w350) -> (0:w347:errorcluster, 2:w342:i64, 3:w345:refnum<file>)
                n97 = while {
                  tunnel: w345 -> [w364]
                  shift-right: [w361] -> w348
                  shift-left: w347 -> [w367]
                  tunnel: w344 -> [w353]
                  tunnel: [w360] -> w340 mode=indexing
                  tunnel: [w359] -> w336
                  tunnel: w335 -> [w355]
                  tunnel: w334 -> [w351]
                  stop <- w363 stop-if-true
                  n98 = Read from Binary File(5:T9 {"SampleRate"=-1.0, "TrigDelay"=0.0, "SpecLength"=0.0, "DAQ_Range"=0.0, "Average#"=0, "Position"=[], "Spectrum"=[], "Calibr."=[], "Pressure"=-1.0, "Desp_LaserEnergy"=-1.0, "PI_LaserEnergy"=-1.0, "Voltages Table"=[], "ProcMode"=enum."None", "Threshold"=-1.0, "Comment"="", "TickCount"=0.0, "Time Stamp"=timestamp(0 s since 1904-01-01)} ("Signal Segment"), 8:w367, 9:T6."little-endian" ("byte order (0:big-endian, network order)"), 11:w364) -> (0:w368:errorcluster, 3:w365:refnum<file>)  [unwired: 2 in, 2 out]
                  n99 = property class="Bool (strict)"(reference=w351) -> ("Value"=w352:bool)  [unwired: 1 in, 2 out]
                  n100 = Get File Position(4:w368, 7:w365) -> (0:w361:errorcluster, 2:w360:i64, 3:w359:refnum<file>)
                  n101 = Add(x=i64 0, y=w360) -> (x+y=w354:i64)
                  n102 = Divide(x=w354, y=w353) -> (x/y=w357:dbl)
                  n103 = Less Or Equal?(x=w353, y=w354) -> (x <= y?=w362:bool)
                  n104 = Multiply(x=w357, y=100.0 ("x")) -> (x*y=w356:dbl)
                  n105 = Compound Arithmetic op=OR(w362, w361, w352) -> (w363:bool)
                  n106 = property class="Slide (strict)"(reference=w355, "Value"=w356) -> ()  [unwired: 1 in, 2 out]
                }
                n107 = Array Size(array=w340) -> (size(s)=w339:i32)
                n108 = Decrement(x=w339) -> (x-1=w338:i32)
                n109 = Array Subset(array=w340, index=0, length=w338) -> (w341:i64[])
                n110 = Build Array (concatenate)(w342, w341) -> (w343:i64[])
              }
              frame "DPv31" {
                n111 = Unbundle By Name(w383) -> ("FileSize"=w381:i64)
                n112 = Get File Position(4:w386, 7:w387) -> (0:w384:errorcluster, 2:w379:i64, 3:w382:refnum<file>)
                n113 = while {
                  tunnel: w382 -> [w402]
                  shift-right: [w399] -> w385
                  shift-left: w384 -> [w405]
                  tunnel: w381 -> [w392]
                  tunnel: [w398] -> w377 mode=indexing
                  tunnel: [w397] -> w373
                  tunnel: w372 -> [w390]
                  tunnel: w371 -> [w389]
                  stop <- w401 stop-if-true
                  n114 = Read from Binary File(5:T10 {"Average#"=0, "SpecLength"=0, "Spectrum"=[], "Cali."=[], "Sample Rate"=0.0} ("cluster"), 8:w405, 9:T6."little-endian" ("byte order (0:big-endian, network order)"), 11:w402) -> (0:w406:errorcluster, 3:w403:refnum<file>)  [unwired: 2 in, 2 out]
                  n115 = property class="Bool (strict)"(reference=w389) -> ("Value"=w388:bool)  [unwired: 1 in, 2 out]
                  n116 = Get File Position(4:w406, 7:w403) -> (0:w399:errorcluster, 2:w398:i64, 3:w397:refnum<file>)
                  n117 = Add(x=i64 0, y=w398) -> (x+y=w393:i64)
                  n118 = Divide(x=w393, y=w392) -> (x/y=w394:dbl)
                  n119 = Less Or Equal?(x=w392, y=w393) -> (x <= y?=w400:bool)
                  n120 = Multiply(x=w394, y=100.0 ("x")) -> (x*y=w391:dbl)
                  n121 = Compound Arithmetic op=OR(w400, w399, w388) -> (w401:bool)
                  n122 = property class="Slide (strict)"(reference=w390, "Value"=w391) -> ()  [unwired: 1 in, 2 out]
                }
                n123 = Array Size(array=w377) -> (size(s)=w376:i32)
                n124 = Decrement(x=w376) -> (x-1=w375:i32)
                n125 = Array Subset(array=w377, index=0, length=w375) -> (w378:i64[])
                n126 = Build Array (concatenate)(w379, w378) -> (w380:i64[])
              }
            }
          }
          frame "Read_i" {
            n127 = Unbundle By Name(w409) -> ("ForceQuit"=w408:refnum<vi>)
            n128 = Unbundle By Name(w418) -> ("FileVersion"=w417:string)
            n129 = case shown="\"YCv36\", Default" w417 {
              tunnel: w419 -> [w435 w500 w565 w614]
              tunnel: w420 -> [w441 w506 w571 w624]
              tunnel: [w424 w489 w554 w607] -> w410
              tunnel: [w425 w490 w555 w619] -> w422
              tunnel: [w440 w505 w570 w622] -> w421
              tunnel: w418 -> [w440 w505 w570 w622]
              tunnel: [w438 w503 w568 w617] -> w416
              tunnel: w415 -> [w438 w503 w568 w617]
              tunnel: w414 -> [w436 w501 w566 w615]
              tunnel: w413 -> [w430 w495 w560 w612]
              tunnel: w412 -> [_ _ _ _]
              tunnel: [w432 w497 w562 w609] -> w411
              tunnel: w408 -> [w423 w488 w553 w606]
              frame "YCv30", "YCv31" {
                n130 = Variant To Data(error in=w435, type=cluster{"index":i32, "length":i32} {"index"=0, "length"=1}, Variant=w436) -> (data=w437:cluster{"index":i32, "length":i32}, error out=w434:errorcluster)
                n131 = Unbundle By Name(w437) -> ("length"=w426:i32, "index"=w433:i32)
                n132 = Index Array(array=w438, index=w433) -> (element=w439:i64)
                n133 = Unbundle By Name(w440) -> ("FileSize"=w427:i64)
                n134 = Set File Position(offset (in bytes) (0)=w439, refnum=w441, error in=w434) -> (refnum out=w429:refnum<file>, error out=w428:errorcluster)  [unwired: 1 in]
                n135 = Add(x=w426, y=w433) -> (x+y=w432:i32)
                n136 = for {
                  N: w426 -> [w472]
                  tunnel: w429 -> [w482]
                  shift-right: [w462] -> w424
                  shift-left: w428 -> [w486]
                  tunnel: w427 -> [w481]
                  tunnel: [w479] -> w425
                  tunnel: w430 -> [w478]
                  tunnel: w423 -> [w449]
                  i -> [w471]
                  stop <- w464 stop-if-true
                  w474 = 1 items=["no exception", "cancel error on match", "set error on match"] ("[exception action] (none:0)")
                  w475 = T15 0 items=["no dialog", "OK message", "continue or stop message", "OK message + warnings", "continue/stop + warnings"] ("type of dialog (OK msg:1)")
                  n137 = Read from Binary File(5:T5 {"Signal"=[], "Calibr."=[], "Position"=[], "Pressure"=0.0, "Desp_LaserEnergy"=0.05, "PI_LaserEnergy"=0.05, "Depth"=0.0, "Average"=0, "Acqu. Rate"=0.0, "Voltages Table"=[], "Acqu. Range"=0.0, "Processing Mode"=enum."None", "Threshold"=0.05, "Comment"="", "Time Stamp"=timestamp(0 s since 1904-01-01), "Operator"=""} ("Signal Segment"), 8:w486, 9:T6."little-endian" ("byte order (0:big-endian, network order)"), 11:w482) -> (0:w477:errorcluster, 2:w457:T5, 3:w483:refnum<file>)  [unwired: 2 in, 1 out]
                  n138 = call <vilib>:"General Error Handler.vi"("type of dialog (OK msg:1)"=w475, "error in (no error)"=w477, "[exception action] (none:0)"=w474, "[exception code]"=116) -> ("error out"=w476:errorcluster)  [unwired: 7 in, 4 out]
                  n139 = property on="ForceQuit" class="Bool (strict)"(reference=w449) -> ("Value"=w450:bool)  [unwired: 1 in, 2 out]
                  n140 = Get File Position(4:w476, 7:w483) -> (0:w461:errorcluster, 2:w480:i64, 3:w479:refnum<file>)
                  n141 = Add(x=i64 0, y=w480) -> (x+y=w485:i64)
                  n142 = Increment(x=w471) -> (x+1=w470:i32)
                  n143 = Less Or Equal?(x=w481, y=w485) -> (x <= y?=w466:bool)
                  n144 = Unbundle By Name(w457) -> ("Acqu. Rate"=w452:dbl, "Depth"=w453:dbl, "Position"=w454:dbl[], "Signal"=w455:sgl[], "Calibr."=w456:dbl[], "Desp_LaserEnergy"=w451:dbl, "PI_LaserEnergy"=w448:dbl, "Average"=w447:i32, "Voltages Table"=w446:sgl[][], "Acqu. Range"=w445:dbl, "Processing Mode"=w444:T3, "Threshold"=w443:dbl, "Time Stamp"=w442:timestamp)
                  n145 = Equal?(x=w472, y=w470) -> (x = y?=w465:bool)
                  n146 = Compound Arithmetic op=OR(w450, w466, w465) -> (w463:bool)
                  n147 = Select(t="End" ("Comment"), s=w463, f="") -> (s? t:f=w469:string)
                  n148 = Bundle By Name(cluster=T11 {"SampleRate"=0.0, "TrigDelay"=0.0, "SpecLength"=0.0, "DAQ_Range"=0.0, "Average#"=0, "Position"=[], "Spectrum"=[], "Calibr."=[], "Pressure"=0.0, "Desp_LaserEnergy"=0.0, "PI_LaserEnergy"=0.0, "Voltages Table"=[], "ProcMode"=enum."None", "Threshold"=0.0, "Comment"="", "TickCount"=0.0, "Time Stamp"=timestamp(0 s since 1904-01-01)} ("Signal Segment"), "Comment"=w469, "SampleRate"=w452, "SpecLength"=w453, "Position"=w454, "Spectrum"=w455, "Calibr."=w456, "Desp_LaserEnergy"=w451, "PI_LaserEnergy"=w448, "Average#"=w447, "Voltages Table"=w446, "DAQ_Range"=w445, "ProcMode"=w444, "Threshold"=w443, "Time Stamp"=w442) -> (w459:T11)
                  n149 = Enqueue Element(queue=w478, element=w459, error in (no error)=w461) -> (error out=w462:errorcluster)  [unwired: 1 in, 2 out]
                  n150 = Or(x=w463, y=w462) -> (x .or. y?=w464:bool)
                }
              }
              frame "YCv35" {
                n151 = Variant To Data(error in=w500, type=cluster{"index":i32, "length":i32} {"index"=0, "length"=1}, Variant=w501) -> (data=w502:cluster{"index":i32, "length":i32}, error out=w499:errorcluster)
                n152 = Unbundle By Name(w502) -> ("length"=w491:i32, "index"=w498:i32)
                n153 = Index Array(array=w503, index=w498) -> (element=w504:i64)
                n154 = Unbundle By Name(w505) -> ("FileSize"=w492:i64)
                n155 = Set File Position(offset (in bytes) (0)=w504, refnum=w506, error in=w499) -> (refnum out=w494:refnum<file>, error out=w493:errorcluster)  [unwired: 1 in]
                n156 = Add(x=w491, y=w498) -> (x+y=w497:i32)
                n157 = for {
                  N: w491 -> [w537]
                  tunnel: w494 -> [w547]
                  shift-right: [w528] -> w489
                  shift-left: w493 -> [w551]
                  tunnel: w492 -> [w546]
                  tunnel: [w544] -> w490
                  tunnel: w495 -> [w543]
                  tunnel: w488 -> [w524]
                  i -> [w536]
                  stop <- w530 stop-if-true
                  w539 = 1 items=["no exception", "cancel error on match", "set error on match"] ("[exception action] (none:0)")
                  w540 = T15 0 items=["no dialog", "OK message", "continue or stop message", "OK message + warnings", "continue/stop + warnings"] ("type of dialog (OK msg:1)")
                  n158 = Read from Binary File(5:T8 {"SampleRate"=0.0, "TrigDelay"=0.0, "SpecLength"=0.0, "DAQ_Range"=0.0, "Average#"=0, "Position"=[], "Spectrum"=[], "Calibr."=[], "Pressure"=0.0, "Desp_LaserEnergy"=0.0, "PI_LaserEnergy"=0.0, "Voltages Table"=[], "ProcMode"=enum."None", "Threshold"=0.0, "Comment"="", "Time Stamp"=timestamp(0 s since 1904-01-01)} ("Signal Segment"), 8:w551, 9:T6."little-endian" ("byte order (0:big-endian, network order)"), 11:w547) -> (0:w542:errorcluster, 2:w507:T8, 3:w548:refnum<file>)  [unwired: 2 in, 1 out]
                  n159 = call <vilib>:"General Error Handler.vi"("type of dialog (OK msg:1)"=w540, "error in (no error)"=w542, "[exception action] (none:0)"=w539, "[exception code]"=116) -> ("error out"=w541:errorcluster)  [unwired: 7 in, 4 out]
                  n160 = property on="ForceQuit" class="Bool (strict)"(reference=w524) -> ("Value"=w525:bool)  [unwired: 1 in, 2 out]
                  n161 = Get File Position(4:w541, 7:w548) -> (0:w527:errorcluster, 2:w545:i64, 3:w544:refnum<file>)
                  n162 = Add(x=i64 0, y=w545) -> (x+y=w550:i64)
                  n163 = Increment(x=w536) -> (x+1=w535:i32)
                  n164 = Less Or Equal?(x=w546, y=w550) -> (x <= y?=w532:bool)
                  n165 = Unbundle By Name(w507) -> ("SampleRate"=w518:dbl, "SpecLength"=w519:dbl, "Position"=w520:dbl[], "Spectrum"=w521:sgl[], "Calibr."=w522:dbl[], "Desp_LaserEnergy"=w517:dbl, "PI_LaserEnergy"=w516:dbl, "Average#"=w515:i32, "Voltages Table"=w514:sgl[][], "PI_LaserEnergy"=w513:dbl, "ProcMode"=w512:T3, "Threshold"=w511:dbl, "Time Stamp"=w510:timestamp)
                  n166 = Equal?(x=w537, y=w535) -> (x = y?=w531:bool)
                  n167 = Compound Arithmetic op=OR(w525, w532, w531) -> (w529:bool)
                  n168 = Select(t="End" ("Comment"), s=w529, f="") -> (s? t:f=w509:string)
                  n169 = Bundle By Name(cluster=T11 {"SampleRate"=0.0, "TrigDelay"=0.0, "SpecLength"=0.0, "DAQ_Range"=0.0, "Average#"=0, "Position"=[], "Spectrum"=[], "Calibr."=[], "Pressure"=0.0, "Desp_LaserEnergy"=0.0, "PI_LaserEnergy"=0.0, "Voltages Table"=[], "ProcMode"=enum."None", "Threshold"=0.0, "Comment"="", "TickCount"=0.0, "Time Stamp"=timestamp(0 s since 1904-01-01)} ("Signal Segment"), "Comment"=w509, "SampleRate"=w518, "SpecLength"=w519, "Position"=w520, "Spectrum"=w521, "Calibr."=w522, "Desp_LaserEnergy"=w517, "PI_LaserEnergy"=w516, "Average#"=w515, "Voltages Table"=w514, "DAQ_Range"=w513, "ProcMode"=w512, "Threshold"=w511, "Time Stamp"=w510) -> (w508:T11)
                  n170 = Enqueue Element(queue=w543, element=w508, error in (no error)=w527) -> (error out=w528:errorcluster)  [unwired: 1 in, 2 out]
                  n171 = Or(x=w529, y=w528) -> (x .or. y?=w530:bool)
                }
              }
              frame "YCv36", Default {
                n172 = Variant To Data(error in=w565, type=cluster{"index":i32, "length":i32} {"index"=0, "length"=1}, Variant=w566) -> (data=w567:cluster{"index":i32, "length":i32}, error out=w564:errorcluster)
                n173 = Unbundle By Name(w567) -> ("length"=w556:i32, "index"=w563:i32)
                n174 = Index Array(array=w568, index=w563) -> (element=w569:i64)
                n175 = Unbundle By Name(w570) -> ("FileSize"=w557:i64)
                n176 = Set File Position(offset (in bytes) (0)=w569, refnum=w571, error in=w564) -> (refnum out=w559:refnum<file>, error out=w558:errorcluster)  [unwired: 1 in]
                n177 = Add(x=w556, y=w563) -> (x+y=w562:i32)
                n178 = for {
                  N: w556 -> [w590]
                  tunnel: w559 -> [w600]
                  shift-right: [w581] -> w554
                  shift-left: w558 -> [w604]
                  tunnel: w557 -> [w599]
                  tunnel: [w597] -> w555
                  tunnel: w560 -> [w596]
                  tunnel: w553 -> [w577]
                  i -> [w589]
                  stop <- w583 stop-if-true
                  w592 = 1 items=["no exception", "cancel error on match", "set error on match"] ("[exception action] (none:0)")
                  w593 = T15 0 items=["no dialog", "OK message", "continue or stop message", "OK message + warnings", "continue/stop + warnings"] ("type of dialog (OK msg:1)")
                  n179 = Read from Binary File(5:T11 {"SampleRate"=-1.0, "TrigDelay"=0.0, "SpecLength"=0.0, "DAQ_Range"=0.0, "Average#"=0, "Position"=[], "Spectrum"=[], "Calibr."=[], "Pressure"=-1.0, "Desp_LaserEnergy"=-1.0, "PI_LaserEnergy"=-1.0, "Voltages Table"=[], "ProcMode"=enum."None", "Threshold"=-1.0, "Comment"="", "TickCount"=0.0, "Time Stamp"=timestamp(0 s since 1904-01-01)} ("Signal Segment"), 8:w604, 9:T6."little-endian" ("byte order (0:big-endian, network order)"), 11:w600) -> (0:w595:errorcluster, 2:w575:T11, 3:w601:refnum<file>)  [unwired: 2 in, 1 out]
                  n180 = call <vilib>:"General Error Handler.vi"("type of dialog (OK msg:1)"=w593, "error in (no error)"=w595, "[exception action] (none:0)"=w592, "[exception code]"=116) -> ("error out"=w594:errorcluster)  [unwired: 7 in, 4 out]
                  n181 = property on="ForceQuit" class="Bool (strict)"(reference=w577) -> ("Value"=w578:bool)  [unwired: 1 in, 2 out]
                  n182 = Get File Position(4:w594, 7:w601) -> (0:w580:errorcluster, 2:w598:i64, 3:w597:refnum<file>)
                  n183 = Add(x=i64 0, y=w598) -> (x+y=w603:i64)
                  n184 = Unbundle By Name(w575) -> ("Comment"=w574:string)
                  n185 = Increment(x=w589) -> (x+1=w588:i32)
                  n186 = Less Or Equal?(x=w599, y=w603) -> (x <= y?=w585:bool)
                  n187 = Equal?(x=w590, y=w588) -> (x = y?=w584:bool)
                  n188 = Compound Arithmetic op=OR(w578, w585, w584) -> (w582:bool)
                  n189 = Select(t="End" ("Comment"), s=w582, f="") -> (s? t:f=w572:string)
                  n190 = Concatenate Strings(w574, w572) -> (w573:string)
                  n191 = Bundle By Name(cluster=w575, "Comment"=w573) -> (w576:T11)
                  n192 = Enqueue Element(queue=w596, element=w576, error in (no error)=w580) -> (error out=w581:errorcluster)  [unwired: 1 in, 2 out]
                  n193 = Or(x=w582, y=w581) -> (x .or. y?=w583:bool)
                }
              }
              frame "DPv31" {
                n194 = Variant To Data(error in=w614, type=cluster{"index":i32, "length":i32} {"index"=0, "length"=1}, Variant=w615) -> (data=w616:cluster{"index":i32, "length":i32}, error out=w613:errorcluster)
                n195 = Unbundle By Name(w616) -> ("length"=w611:i32, "index"=w610:i32)
                n196 = Index Array(array=w617, index=w610) -> (element=w618:i64)
                n197 = Unbundle By Name(w622) -> ("FileSize"=w620:i64)
                n198 = Set File Position(offset (in bytes) (0)=w618, refnum=w624, error in=w613) -> (refnum out=w621:refnum<file>, error out=w623:errorcluster)  [unwired: 1 in]
                n199 = Add(x=w611, y=w610) -> (x+y=w609:i32)
                n200 = for {
                  N: w611 -> [w638]
                  tunnel: w621 -> [w657]
                  shift-right: [w628] -> w607
                  shift-left: w623 -> [w661]
                  tunnel: w620 -> [w656]
                  tunnel: [w654] -> w619
                  tunnel: w612 -> [w653]
                  tunnel: w606 -> [w625]
                  i -> [w637]
                  stop <- w630 stop-if-true
                  w649 = 1 items=["no exception", "cancel error on match", "set error on match"] ("[exception action] (none:0)")
                  w650 = T15 0 items=["no dialog", "OK message", "continue or stop message", "OK message + warnings", "continue/stop + warnings"] ("type of dialog (OK msg:1)")
                  n201 = Read from Binary File(5:T10 {"Average#"=0, "SpecLength"=0, "Spectrum"=[], "Cali."=[], "Sample Rate"=0.0} ("cluster"), 8:w661, 9:T6."little-endian" ("byte order (0:big-endian, network order)"), 11:w657) -> (0:w652:errorcluster, 2:w645:T10, 3:w658:refnum<file>)  [unwired: 2 in, 1 out]
                  n202 = call <vilib>:"General Error Handler.vi"("type of dialog (OK msg:1)"=w650, "error in (no error)"=w652, "[exception action] (none:0)"=w649, "[exception code]"=116) -> ("error out"=w651:errorcluster)  [unwired: 7 in, 4 out]
                  n203 = property on="ForceQuit" class="Bool (strict)"(reference=w625) -> ("Value"=w626:bool)  [unwired: 1 in, 2 out]
                  n204 = Get File Position(4:w651, 7:w658) -> (0:w627:errorcluster, 2:w655:i64, 3:w654:refnum<file>)
                  n205 = Add(x=i64 0, y=w655) -> (x+y=w660:i64)
                  n206 = Increment(x=w637) -> (x+1=w636:i32)
                  n207 = Less Or Equal?(x=w656, y=w660) -> (x <= y?=w632:bool)
                  n208 = Equal?(x=w638, y=w636) -> (x = y?=w631:bool)
                  n209 = Unbundle By Name(w645) -> ("Spectrum"=w644:sgl[], "Cali."=w643:dbl[], "SpecLength"=w642:i32, "Average#"=w641:i16, "Sample Rate"=w640:dbl)
                  n210 = Compound Arithmetic op=OR(w626, w632, w631) -> (w629:bool)
                  n211 = Select(t="End" ("Comment"), s=w629, f="") -> (s? t:f=w635:string)
                  n212 = Bundle By Name(cluster=T11 {"SampleRate"=0.0, "TrigDelay"=0.0, "SpecLength"=0.0, "DAQ_Range"=0.0, "Average#"=0, "Position"=[], "Spectrum"=[], "Calibr."=[], "Pressure"=0.0, "Desp_LaserEnergy"=0.0, "PI_LaserEnergy"=0.0, "Voltages Table"=[], "ProcMode"=enum."None", "Threshold"=0.0, "Comment"="", "TickCount"=0.0, "Time Stamp"=timestamp(0 s since 1904-01-01)} ("Signal Segment"), "Comment"=w635, "Spectrum"=w644, "Calibr."=w643, "SpecLength"=w642, "Average#"=w641, "SampleRate"=w640) -> (w646:T11)
                  n213 = Enqueue Element(queue=w653, element=w646, error in (no error)=w627) -> (error out=w628:errorcluster)  [unwired: 1 in, 2 out]
                  n214 = Or(x=w629, y=w628) -> (x .or. y?=w630:bool)
                }
              }
            }
          }
          frame "Read_all" {
            n215 = Unbundle By Name(w666) -> ("Percentage"=w665:refnum<vi>, "ForceQuit"=w664:refnum<vi>)
            n216 = Unbundle By Name(w670) -> ("FileVersion"=w669:string)
            n217 = case shown="\"YCv36\", Default" w669 {
              tunnel: w671 -> [w692 w751 w810 w887]
              tunnel: w672 -> [w693 w752 w811 w888]
              tunnel: [w691 w750 w809 w886] -> w675
              tunnel: [w679 w738 w797 w874] -> w674
              tunnel: [w689 w748 w807 w884] -> w673
              tunnel: w670 -> [w689 w748 w807 w884]
              tunnel: [w686 w745 w804 w881] -> w668
              tunnel: w665 -> [w678 w737 w796 w873]
              tunnel: w664 -> [w677 w736 w795 w872]
              tunnel: w663 -> [w676 w735 w794 _]
              frame "YCv30", "YCv31" {
                n218 = Unbundle By Name(w689) -> ("FileSize"=w687:i64)
                n219 = Get File Position(4:w692, 7:w693) -> (0:w690:errorcluster, 2:w685:i64, 3:w688:refnum<file>)
                n220 = while {
                  tunnel: w688 -> [w728]
                  shift-right: [w695] -> w691
                  shift-left: w690 -> [w731]
                  tunnel: w687 -> [w719]
                  tunnel: [w726] -> w683 mode=indexing
                  tunnel: [w725] -> w679
                  tunnel: w678 -> [w721]
                  tunnel: w677 -> [w717]
                  tunnel: w676 -> [w697]
                  stop <- w694 stop-if-true
                  n221 = Read from Binary File(5:T5 {"Signal"=[], "Calibr."=[], "Position"=[], "Pressure"=0.0, "Desp_LaserEnergy"=0.05, "PI_LaserEnergy"=0.05, "Depth"=0.0, "Average"=0, "Acqu. Rate"=0.0, "Voltages Table"=[], "Acqu. Range"=0.0, "Processing Mode"=enum."None", "Threshold"=0.05, "Comment"="", "Time Stamp"=timestamp(0 s since 1904-01-01), "Operator"=""} ("Signal Segment"), 8:w731, 9:T6."little-endian" ("byte order (0:big-endian, network order)"), 11:w728) -> (0:w732:errorcluster, 2:w699:T5, 3:w729:refnum<file>)  [unwired: 2 in, 1 out]
                  n222 = property class="Bool (strict)"(reference=w717) -> ("Value"=w718:bool)  [unwired: 1 in, 2 out]
                  n223 = Get File Position(4:w732, 7:w729) -> (0:w696:errorcluster, 2:w726:i64, 3:w725:refnum<file>)
                  n224 = Add(x=i64 0, y=w726) -> (x+y=w720:i64)
                  n225 = Divide(x=w720, y=w719) -> (x/y=w723:dbl)
                  n226 = Less Or Equal?(x=w719, y=w720) -> (x <= y?=w727:bool)
                  n227 = Unbundle By Name(w699) -> ("Acqu. Rate"=w708:dbl, "Depth"=w709:dbl, "Position"=w710:dbl[], "Signal"=w711:sgl[], "Calibr."=w712:dbl[], "Desp_LaserEnergy"=w707:dbl, "PI_LaserEnergy"=w706:dbl, "Average"=w705:i32, "Voltages Table"=w704:sgl[][], "Acqu. Range"=w703:dbl, "Processing Mode"=w702:T3, "Threshold"=w701:dbl, "Time Stamp"=w700:timestamp)
                  n228 = Multiply(x=w723, y=100.0 ("x")) -> (x*y=w722:dbl)
                  n229 = Compound Arithmetic op=OR(w727, w696, w718) -> (w694:bool)
                  n230 = property on="Percentage" class="Slide (strict)"(reference=w721, "Value"=w722) -> ()  [unwired: 1 in, 2 out]
                  n231 = Select(t="End" ("Comment"), s=w694, f="") -> (s? t:f=w716:string)
                  n232 = Bundle By Name(cluster=T11 {"SampleRate"=0.0, "TrigDelay"=0.0, "SpecLength"=0.0, "DAQ_Range"=0.0, "Average#"=0, "Position"=[], "Spectrum"=[], "Calibr."=[], "Pressure"=0.0, "Desp_LaserEnergy"=0.0, "PI_LaserEnergy"=0.0, "Voltages Table"=[], "ProcMode"=enum."None", "Threshold"=0.0, "Comment"="", "TickCount"=0.0, "Time Stamp"=timestamp(0 s since 1904-01-01)} ("Signal Segment"), "Comment"=w716, "SampleRate"=w708, "SpecLength"=w709, "Position"=w710, "Spectrum"=w711, "Calibr."=w712, "Desp_LaserEnergy"=w707, "PI_LaserEnergy"=w706, "Average#"=w705, "Voltages Table"=w704, "DAQ_Range"=w703, "ProcMode"=w702, "Threshold"=w701, "Time Stamp"=w700) -> (w698:T11)
                  n233 = Enqueue Element(queue=w697, element=w698, error in (no error)=w696) -> (error out=w695:errorcluster)  [unwired: 1 in, 2 out]
                }
                n234 = Array Size(array=w683) -> (size(s)=w682:i32)
                n235 = Decrement(x=w682) -> (x-1=w681:i32)
                n236 = Array Subset(array=w683, index=0, length=w681) -> (w684:i64[])
                n237 = Build Array (concatenate)(w685, w684) -> (w686:i64[])
              }
              frame "YCv35" {
                n238 = Unbundle By Name(w748) -> ("FileSize"=w746:i64)
                n239 = Get File Position(4:w751, 7:w752) -> (0:w749:errorcluster, 2:w744:i64, 3:w747:refnum<file>)
                n240 = while {
                  tunnel: w747 -> [w787]
                  shift-right: [w757] -> w750
                  shift-left: w749 -> [w790]
                  tunnel: w746 -> [w778]
                  tunnel: [w785] -> w742 mode=indexing
                  tunnel: [w784] -> w738
                  tunnel: w737 -> [w780]
                  tunnel: w736 -> [w776]
                  tunnel: w735 -> [w756]
                  stop <- w754 stop-if-true
                  n241 = Read from Binary File(5:T8 {"SampleRate"=-1.0, "TrigDelay"=0.0, "SpecLength"=0.0, "DAQ_Range"=0.0, "Average#"=0, "Position"=[], "Spectrum"=[], "Calibr."=[], "Pressure"=-1.0, "Desp_LaserEnergy"=-1.0, "PI_LaserEnergy"=-1.0, "Voltages Table"=[], "ProcMode"=enum."None", "Threshold"=-1.0, "Comment"="", "Time Stamp"=timestamp(0 s since 1904-01-01)} ("Signal Segment"), 8:w790, 9:T6."little-endian" ("byte order (0:big-endian, network order)"), 11:w787) -> (0:w791:errorcluster, 2:w755:T8, 3:w788:refnum<file>)  [unwired: 2 in, 1 out]
                  n242 = property class="Bool (strict)"(reference=w776) -> ("Value"=w777:bool)  [unwired: 1 in, 2 out]
                  n243 = Get File Position(4:w791, 7:w788) -> (0:w758:errorcluster, 2:w785:i64, 3:w784:refnum<file>)
                  n244 = Add(x=i64 0, y=w785) -> (x+y=w779:i64)
                  n245 = Divide(x=w779, y=w778) -> (x/y=w782:dbl)
                  n246 = Less Or Equal?(x=w778, y=w779) -> (x <= y?=w786:bool)
                  n247 = Multiply(x=w782, y=100.0 ("x")) -> (x*y=w781:dbl)
                  n248 = Unbundle By Name(w755) -> ("Comment"=w753:string, "SampleRate"=w768:dbl, "SpecLength"=w769:dbl, "Position"=w770:dbl[], "Spectrum"=w771:sgl[], "Calibr."=w772:dbl[], "Desp_LaserEnergy"=w767:dbl, "PI_LaserEnergy"=w766:dbl, "Average#"=w765:i32, "Voltages Table"=w764:sgl[][], "PI_LaserEnergy"=w763:dbl, "ProcMode"=w762:T3, "Threshold"=w761:dbl, "Time Stamp"=w760:timestamp)
                  n249 = Compound Arithmetic op=OR(w786, w758, w777) -> (w754:bool)
                  n250 = property class="Slide (strict)"(reference=w780, "Value"=w781) -> ()  [unwired: 1 in, 2 out]
                  n251 = Select(t="End" ("Comment"), s=w754, f=w753) -> (s? t:f=w775:string)
                  n252 = Bundle By Name(cluster=T11 {"SampleRate"=0.0, "TrigDelay"=0.0, "SpecLength"=0.0, "DAQ_Range"=0.0, "Average#"=0, "Position"=[], "Spectrum"=[], "Calibr."=[], "Pressure"=0.0, "Desp_LaserEnergy"=0.0, "PI_LaserEnergy"=0.0, "Voltages Table"=[], "ProcMode"=enum."None", "Threshold"=0.0, "Comment"="", "TickCount"=0.0, "Time Stamp"=timestamp(0 s since 1904-01-01)} ("Signal Segment"), "Comment"=w775, "SampleRate"=w768, "SpecLength"=w769, "Position"=w770, "Spectrum"=w771, "Calibr."=w772, "Desp_LaserEnergy"=w767, "PI_LaserEnergy"=w766, "Average#"=w765, "Voltages Table"=w764, "DAQ_Range"=w763, "ProcMode"=w762, "Threshold"=w761, "Time Stamp"=w760) -> (w759:T11)
                  n253 = Enqueue Element(queue=w756, element=w759, error in (no error)=w758) -> (error out=w757:errorcluster)  [unwired: 1 in, 2 out]
                }
                n254 = Array Size(array=w742) -> (size(s)=w741:i32)
                n255 = Decrement(x=w741) -> (x-1=w740:i32)
                n256 = Array Subset(array=w742, index=0, length=w740) -> (w743:i64[])
                n257 = Build Array (concatenate)(w744, w743) -> (w745:i64[])
              }
              frame "YCv36", Default {
                n258 = Unbundle By Name(w807) -> ("FileSize"=w805:i64)
                n259 = Get File Position(4:w810, 7:w811) -> (0:w808:errorcluster, 2:w803:i64, 3:w806:refnum<file>)
                n260 = while {
                  tunnel: w806 -> [w854]
                  shift-right: [w829] -> w809
                  shift-left: w808 -> [w857]
                  tunnel: [w853] -> w801 mode=indexing
                  tunnel: [w824] -> w797
                  tunnel: w796 -> [w848]
                  tunnel: w795 -> [w845]
                  tunnel: w794 -> [w828]
                  shift-right: [w820] -> _
                  shift-left: w805 -> [w819]
                  stop <- w814 stop-if-true
                  n261 = Read from Binary File(5:T9 {"SampleRate"=-1.0, "TrigDelay"=0.0, "SpecLength"=0.0, "DAQ_Range"=0.0, "Average#"=0, "Position"=[], "Spectrum"=[], "Calibr."=[], "Pressure"=-1.0, "Desp_LaserEnergy"=-1.0, "PI_LaserEnergy"=-1.0, "Voltages Table"=[], "ProcMode"=enum."None", "Threshold"=-1.0, "Comment"="", "TickCount"=0.0, "Time Stamp"=timestamp(0 s since 1904-01-01)} ("Signal Segment"), 8:w857, 9:T6."little-endian" ("byte order (0:big-endian, network order)"), 11:w854) -> (0:w858:errorcluster, 2:w827:T9, 3:w855:refnum<file>)  [unwired: 2 in, 1 out]
                  n262 = Unbundle By Name(w827) -> ("Comment"=w812:string, "SampleRate"=w839:dbl, "SpecLength"=w840:dbl, "Position"=w841:dbl[], "Spectrum"=w842:sgl[], "Calibr."=w843:dbl[], "Desp_LaserEnergy"=w838:dbl, "TickCount"=w826:dbl, "PI_LaserEnergy"=w837:dbl, "Average#"=w836:i32, "Voltages Table"=w835:sgl[][], "PI_LaserEnergy"=w834:dbl, "ProcMode"=w833:T3, "Threshold"=w832:dbl, "Time Stamp"=w831:timestamp, "TickCount"=w825:dbl)
                  n263 = property class="Bool (strict)"(reference=w845) -> ("Value"=w846:bool)  [unwired: 1 in, 2 out]
                  n264 = Get File Position(4:w858, 7:w855) -> (0:w823:errorcluster, 2:w853:i64, 3:w852:refnum<file>)
                  n265 = Add(x=i64 0, y=w853) -> (x+y=w847:i64)
                  n266 = Divide(x=w847, y=w819) -> (x/y=w850:dbl)
                  n267 = Less Or Equal?(x=w819, y=w847) -> (x <= y?=w821:bool)
                  n268 = Multiply(x=w850, y=100.0 ("x")) -> (x*y=w849:dbl)
                  n269 = case "Check if file is still writing." shown="True" w821 {
                    tunnel: w852 -> [w863 w871]
                    tunnel: [w863 w870] -> w824
                    tunnel: w823 -> [w862 w869]
                    tunnel: [w862 w868] -> w822
                    tunnel: [w861 w867] -> w820
                    tunnel: w819 -> [w861 w866]
                    tunnel: [_ w865] -> w818
                    frame False {
                    }
                    frame True {
                      n270 = Get File Size(file=w871, error in=w869) -> (refnum out=w870:refnum<file>, size (in bytes)=w867:i64, 0:w868:errorcluster)
                      n271 = Wait (ms)(milliseconds to wait=u32 1000) -> ()  [unwired: 1 out]
                      n272 = Equal?(x=w867, y=w866) -> (x = y?=w865:bool)
                    }
                  }
                  n273 = Compound Arithmetic op=OR(w818, w823, w846) -> (w814:bool)
                  n274 = property class="Slide (strict)"(reference=w848, "Value"=w849) -> ()  [unwired: 1 in, 2 out]
                  n275 = Select(t="EOF" ("Comment"), s=w814, f="") -> (s? t:f=w815:string)
                  n276 = Concatenate Strings(w812, w815) -> (w813:string)
                  n277 = Bundle By Name(cluster=T11 {"SampleRate"=0.0, "TrigDelay"=0.0, "SpecLength"=0.0, "DAQ_Range"=0.0, "Average#"=0, "Position"=[], "Spectrum"=[], "Calibr."=[], "Pressure"=0.0, "Desp_LaserEnergy"=0.0, "PI_LaserEnergy"=0.0, "Voltages Table"=[], "ProcMode"=enum."None", "Threshold"=0.0, "Comment"="", "TickCount"=0.0, "Time Stamp"=timestamp(0 s since 1904-01-01)} ("Signal Segment"), "Comment"=w813, "SampleRate"=w839, "SpecLength"=w840, "Position"=w841, "Spectrum"=w842, "Calibr."=w843, "Desp_LaserEnergy"=w838, "TickCount"=w826, "PI_LaserEnergy"=w837, "Average#"=w836, "Voltages Table"=w835, "DAQ_Range"=w834, "ProcMode"=w833, "Threshold"=w832, "Time Stamp"=w831, "TickCount"=w825) -> (w830:T11)
                  n278 = Enqueue Element(queue=w828, element=w830, error in (no error)=w822) -> (error out=w829:errorcluster)  [unwired: 1 in, 2 out]
                }
                n279 = Array Size(array=w801) -> (size(s)=w800:i32)
                n280 = Decrement(x=w800) -> (x-1=w799:i32)
                n281 = Array Subset(array=w801, index=0, length=w799) -> (w802:i64[])
                n282 = Build Array (concatenate)(w803, w802) -> (w804:i64[])
              }
              frame "DPv31" {
                n283 = Unbundle By Name(w884) -> ("FileSize"=w882:i64)
                n284 = Get File Position(4:w887, 7:w888) -> (0:w885:errorcluster, 2:w880:i64, 3:w883:refnum<file>)
                n285 = while {
                  tunnel: w883 -> [w903]
                  shift-right: [w900] -> w886
                  shift-left: w885 -> [w906]
                  tunnel: w882 -> [w893]
                  tunnel: [w899] -> w878 mode=indexing
                  tunnel: [w898] -> w874
                  tunnel: w873 -> [w891]
                  tunnel: w872 -> [w890]
                  stop <- w902 stop-if-true
                  n286 = Read from Binary File(5:T10 {"Average#"=0, "SpecLength"=0, "Spectrum"=[], "Cali."=[], "Sample Rate"=0.0} ("cluster"), 8:w906, 9:T6."little-endian" ("byte order (0:big-endian, network order)"), 11:w903) -> (0:w907:errorcluster, 3:w904:refnum<file>)  [unwired: 2 in, 2 out]
                  n287 = property class="Bool (strict)"(reference=w890) -> ("Value"=w889:bool)  [unwired: 1 in, 2 out]
                  n288 = Get File Position(4:w907, 7:w904) -> (0:w900:errorcluster, 2:w899:i64, 3:w898:refnum<file>)
                  n289 = Add(x=i64 0, y=w899) -> (x+y=w894:i64)
                  n290 = Divide(x=w894, y=w893) -> (x/y=w895:dbl)
                  n291 = Less Or Equal?(x=w893, y=w894) -> (x <= y?=w901:bool)
                  n292 = Multiply(x=w895, y=100.0 ("x")) -> (x*y=w892:dbl)
                  n293 = Compound Arithmetic op=OR(w901, w900, w889) -> (w902:bool)
                  n294 = property class="Slide (strict)"(reference=w891, "Value"=w892) -> ()  [unwired: 1 in, 2 out]
                }
                n295 = Array Size(array=w878) -> (size(s)=w877:i32)
                n296 = Decrement(x=w877) -> (x-1=w876:i32)
                n297 = Array Subset(array=w878, index=0, length=w876) -> (w879:i64[])
                n298 = Build Array (concatenate)(w880, w879) -> (w881:i64[])
              }
            }
          }
          frame "Close" {
            n299 = Close File(refnum=w915, error in=w911) -> (error out=w912:errorcluster)  [unwired: 1 out]
            n300 = call <vilib>:"Clear Errors.vi"("error in (no error)"=w912) -> ("error out"=w910:errorcluster)  [unwired: 6 in]
          }
          frame "Quit" {
            n301 = Release Queue(queue=w916) -> ()  [unwired: 2 in, 3 out]
            n302 = Release Queue(queue=w919) -> ()  [unwired: 2 in, 3 out]
            n303 = Release Queue(queue=w917) -> ()  [unwired: 2 in, 3 out]
          }
        }
      }
      frame Error {
      }
    }
  }
